vi "Keyence handler_EIP.vi"(8 "error in (no error)":errorcluster, 11 "Message Queues out":T4) -> (0 "error out":errorcluster, 3 "Message Queue":refnum<queue>)   [LabVIEW 2014]
uses:
  support/Message Queue/Message Queue.lvlib
  support/Message Queue/Enqueue Message (Single).vi
  <vilib>/ErrorRing/Error Ring.xnode
  support/Message Queue/Lossy Enqueue Message (Single).vi
  Keyence data cluster_EIP.ctl
  <vilib>/ethernetip/ethernetip.lvlib
  <vilib>/Utility/error.llb/Error Cluster From Error Code.vi
  <vilib>/ethernetip/ethernetip.llb/ethernetip.ctl
  <vilib>/ethernetip/ethernetip.llb/EthernetIPAssemblyType.ctl
  <vilib>/ethernetip/ethernetip.llb/EthernetIP Tag Write BOOL.vi
  Control_EIP.ctl
  Status_EIP.ctl
  support/Message Queue/Message Cluster.ctl
  support/Message Queue/All Message Queues.ctl
panel:
  in  "Inst 2":i32=1
  in  "Inst":i32=1
  in  "Class":i32=1
  in  "Class 2":i32=1
  in  "Attribute 2":i32=1
  in  "Attribute":i32=1
  out "Keyence Data Cluster":T1
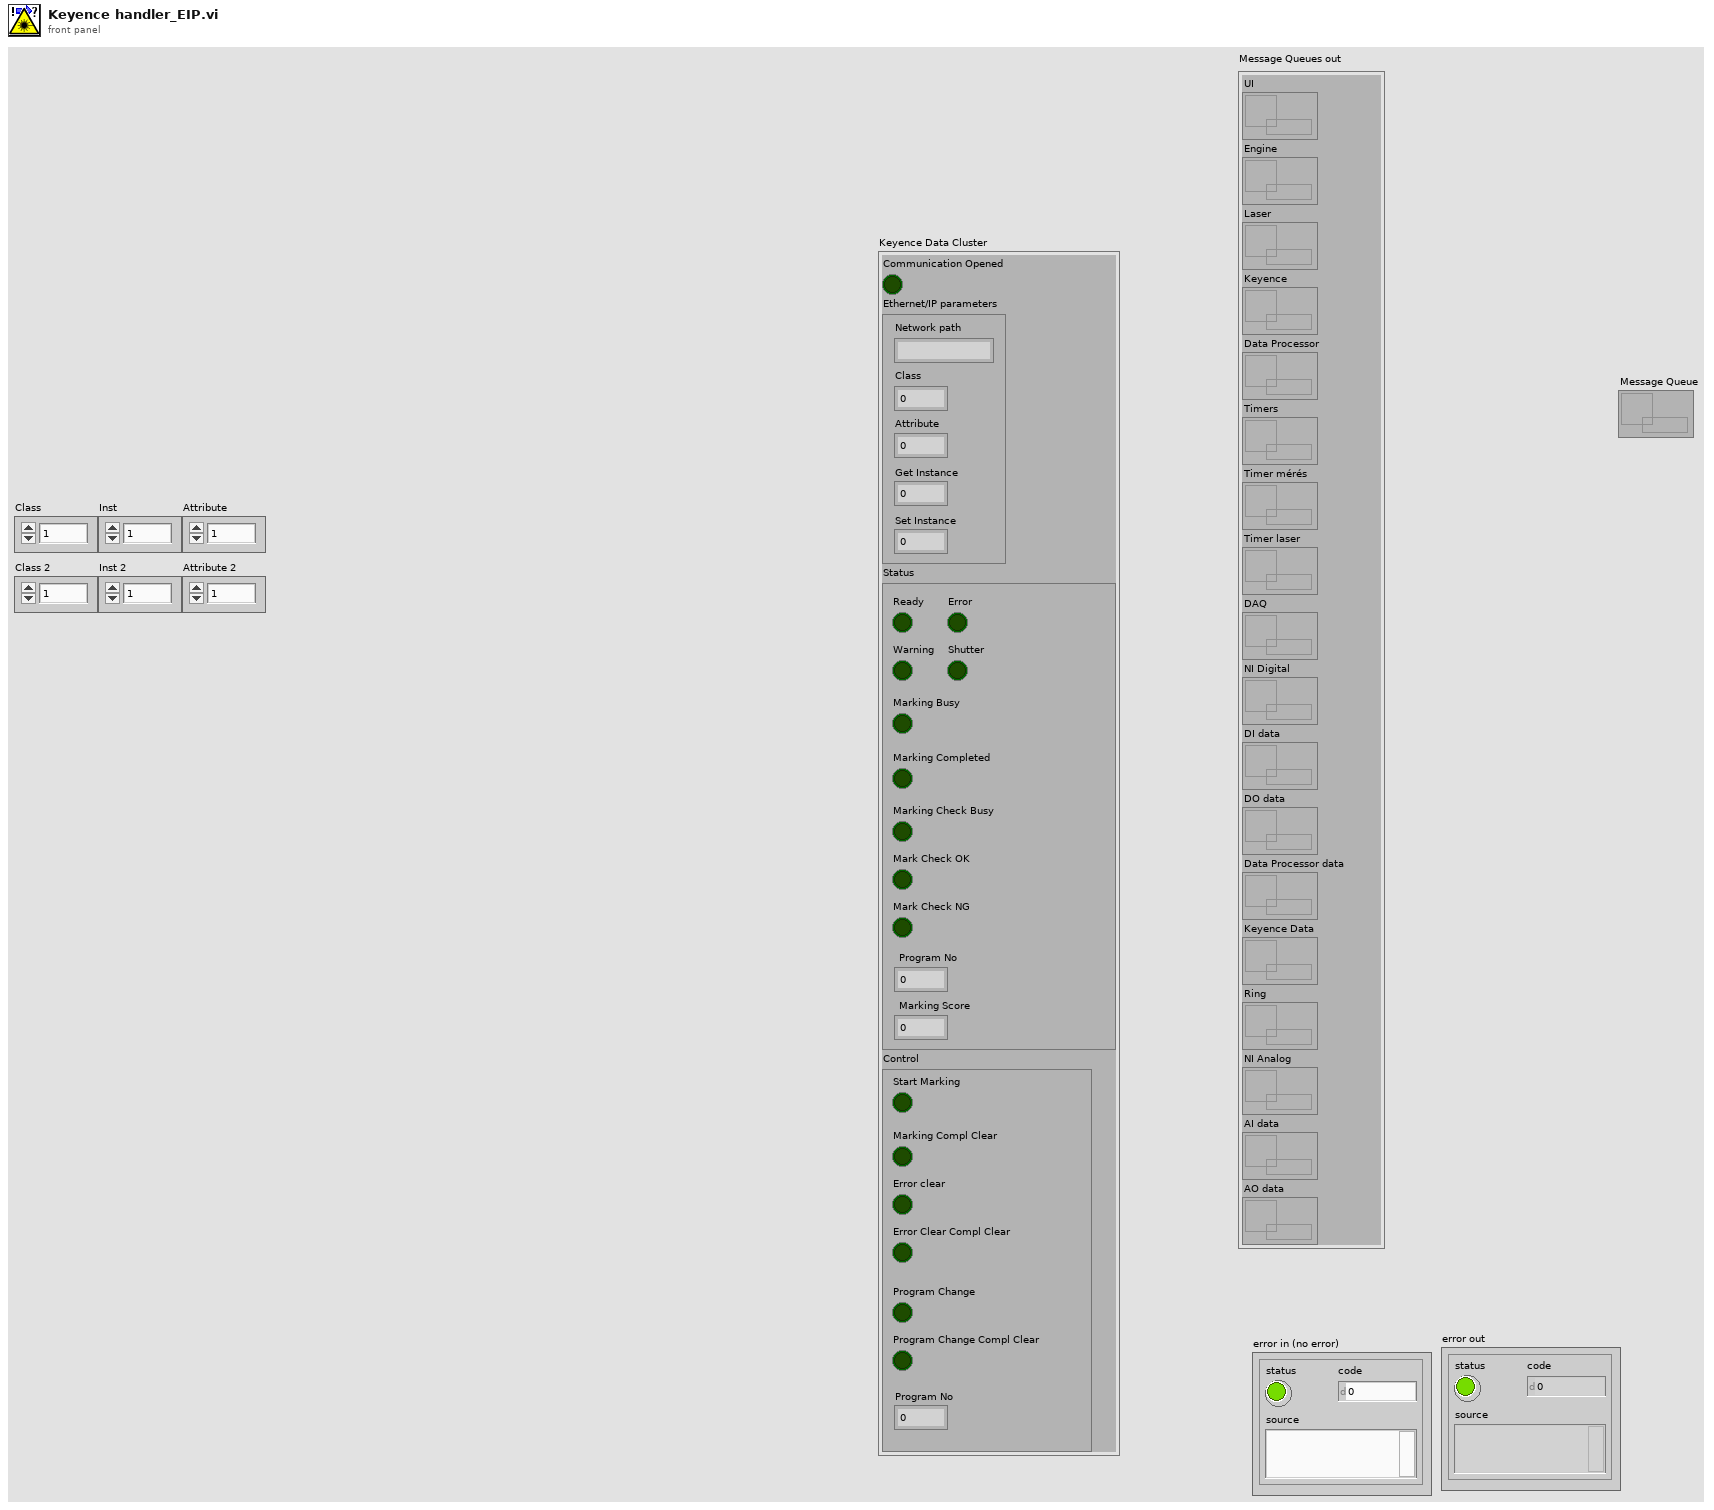
[diagram p1: front panel]
types:
  T1 = typedef "Keyence data cluster_EIP.ctl" = cluster{"Communication Opened":bool, "Ethernet/IP parameters":cluster{"Class":dbl, "Attribute":dbl, "Get Instance":dbl, "Set Instance":dbl, "Network path":string}, "Status":T2, "Control":T3}
  T2 = typedef "Status_EIP.ctl" = cluster{"Ready":bool, "Error":bool, "Warning":bool, "Shutter":bool, "Mark Check OK":bool, "Mark Check NG":bool, "Marking Busy":bool, "Program No":u16, "Marking Check Busy":bool, "Marking Completed":bool, "Marking Score":u16}
  T3 = typedef "Control_EIP.ctl" = cluster{"Start Marking":bool, "Error clear":bool, "Program Change":bool, "Marking Compl Clear":bool, "Program No":u16, "Error Clear Compl Clear":bool, "Program Change Compl Clear":bool}
  T4 = typedef "Message Queue.lvlib/All Message Queues.ctl" = cluster{"UI":refnum<queue>, "Engine":refnum<queue>, "Laser":refnum<queue>, "Keyence":refnum<queue>, "Data Processor":refnum<queue>, "Timers":refnum<queue>, "Timer mérés":refnum<queue>, "Timer laser":refnum<queue>, "DAQ":refnum<queue>, "NI Digital":refnum<queue>, "DI data":refnum<queue>, "DO data":refnum<queue>, "Data Processor data":refnum<queue>, "Keyence Data":refnum<queue>, "Ring":refnum<queue>, "NI Analog":refnum<queue>, "AI data":refnum<queue>, "AO data":refnum<queue>}
  T5 = typedef "ethernetip.lvlib/ethernetip.ctl" = refnum<k21>
  T6 = typedef "ethernetip.lvlib/EthernetIPAssemblyType.ctl" = enum16{"Producing", "Consuming", "Configuration"}
  T7 = typedef "Status.ctl" = cluster{"Ready":bool, "Error":bool, "Warning":bool, "Shutter":bool, "Mark Check OK":bool, "Mark Check NG":bool, "Marking Busy":bool, "Program No":u16, "Marking Check Busy":bool, "Marking Completed":bool, "Marking Score":u16, "Marking Error":bool, "Marking Stop":bool, "Program is changing":bool, "Date/Time":timestamp}
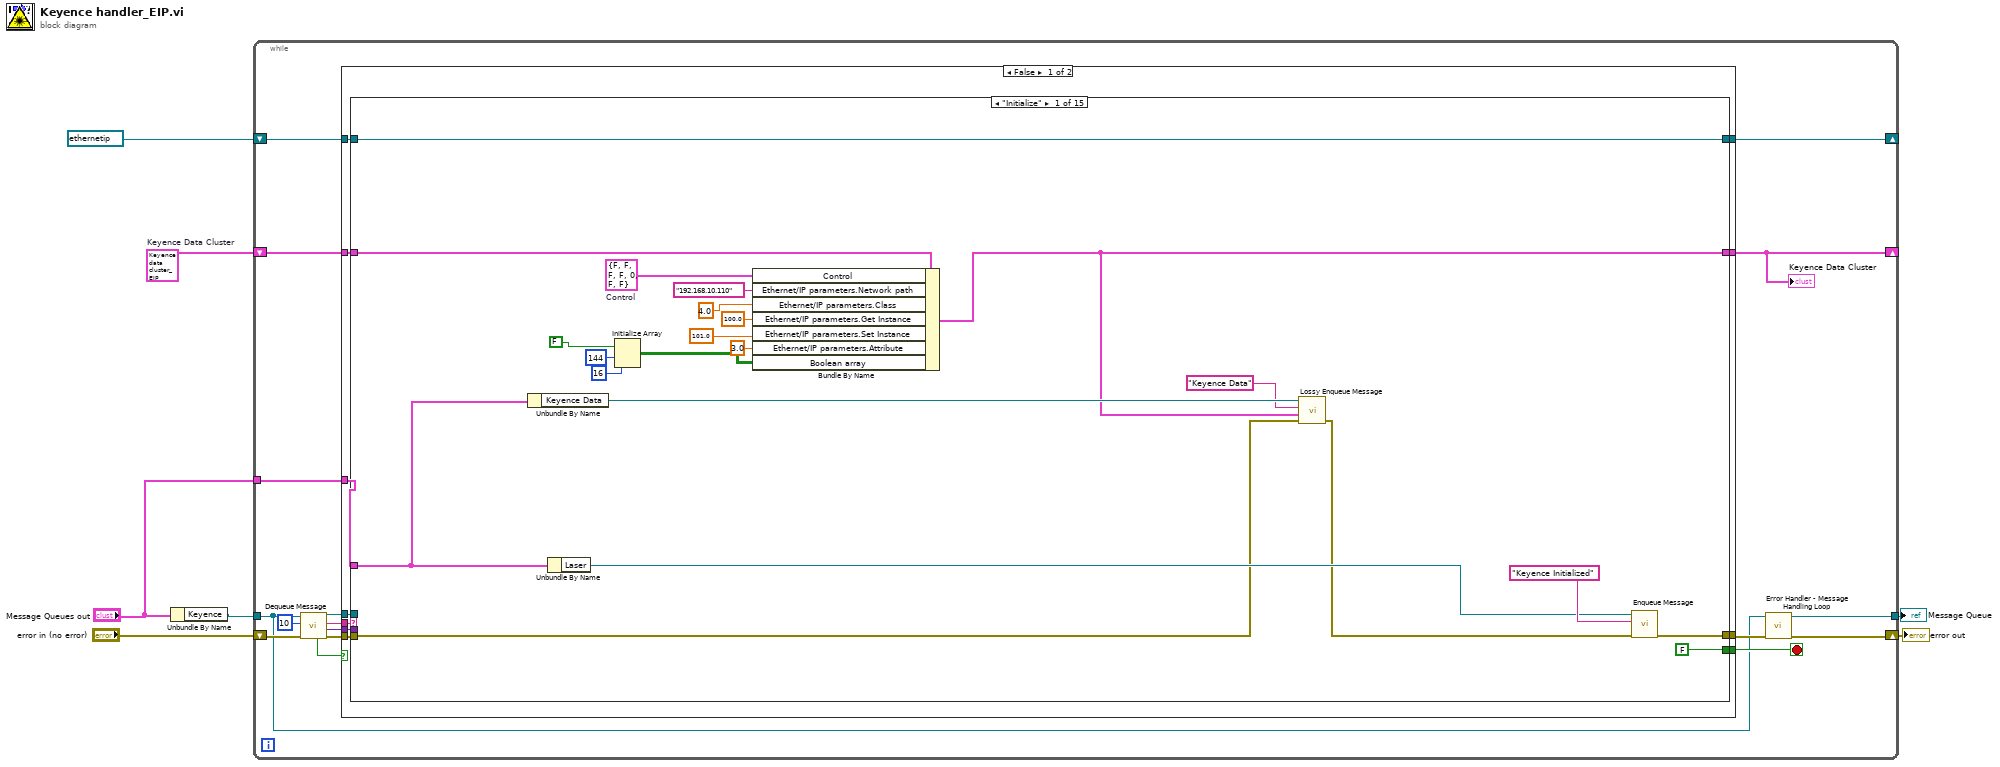
[diagram p0: block diagram]
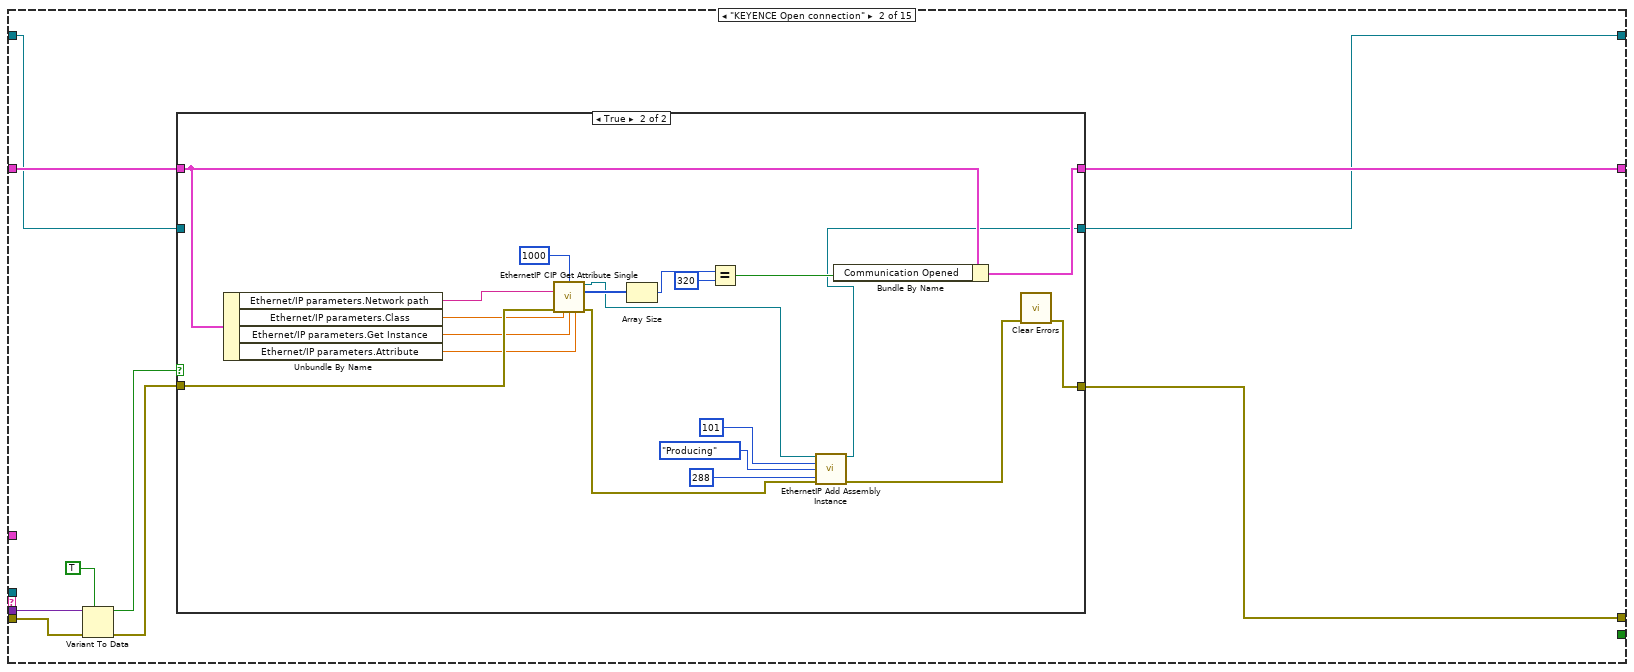
[diagram p2: hidden frame]
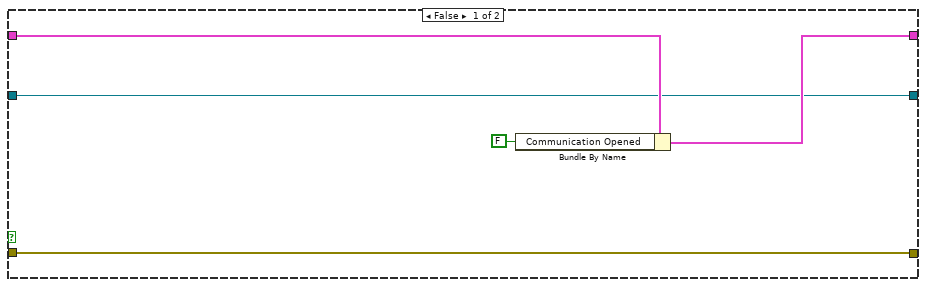
[diagram p3: hidden frame]
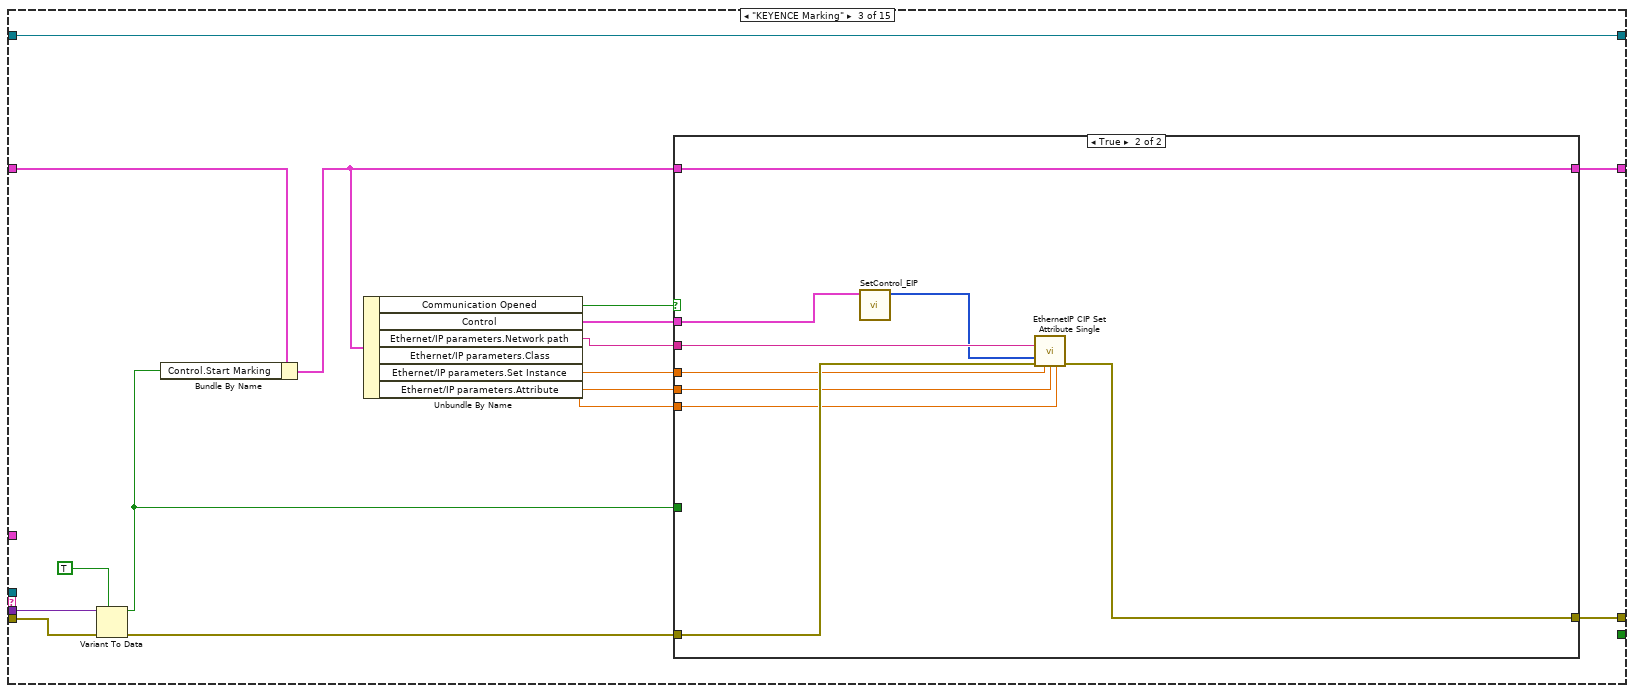
[diagram p4: hidden frame]
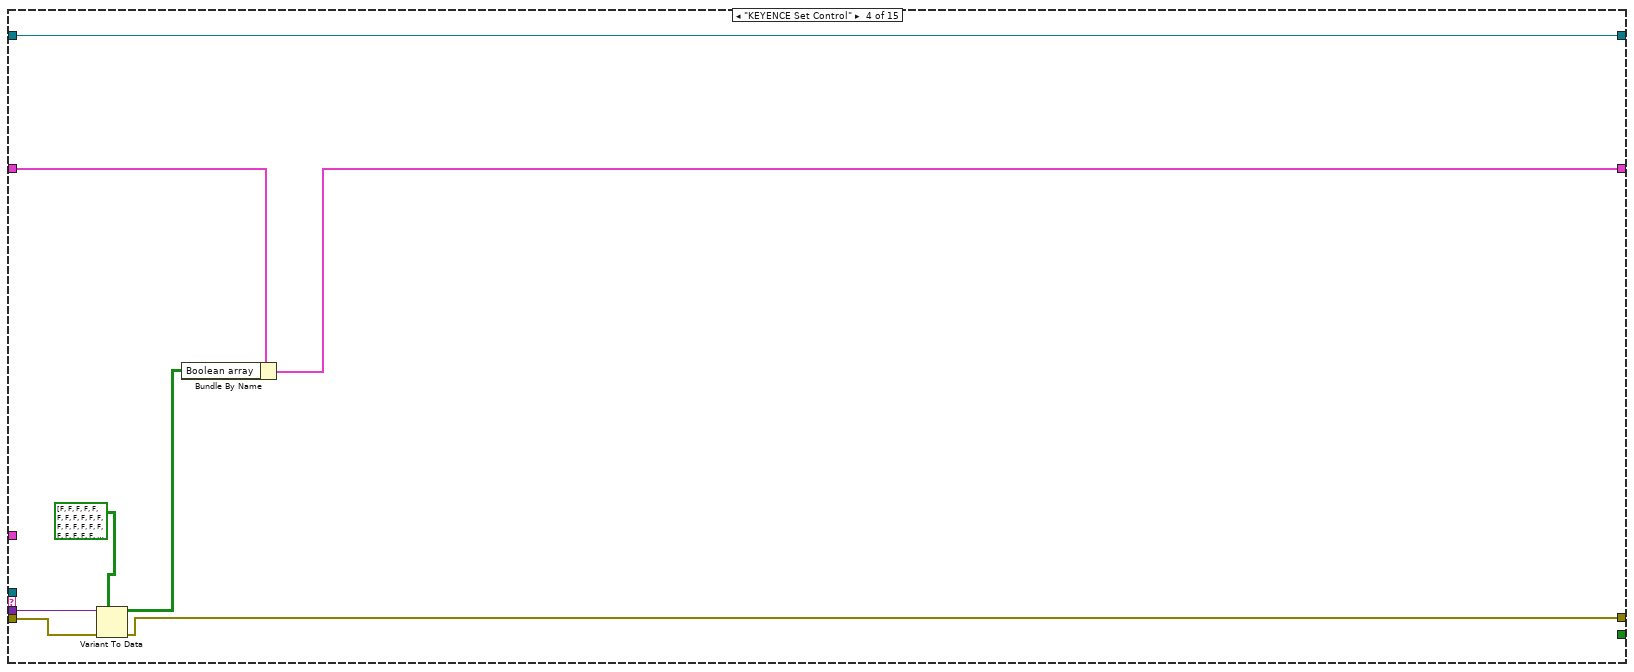
[diagram p6: hidden frame]
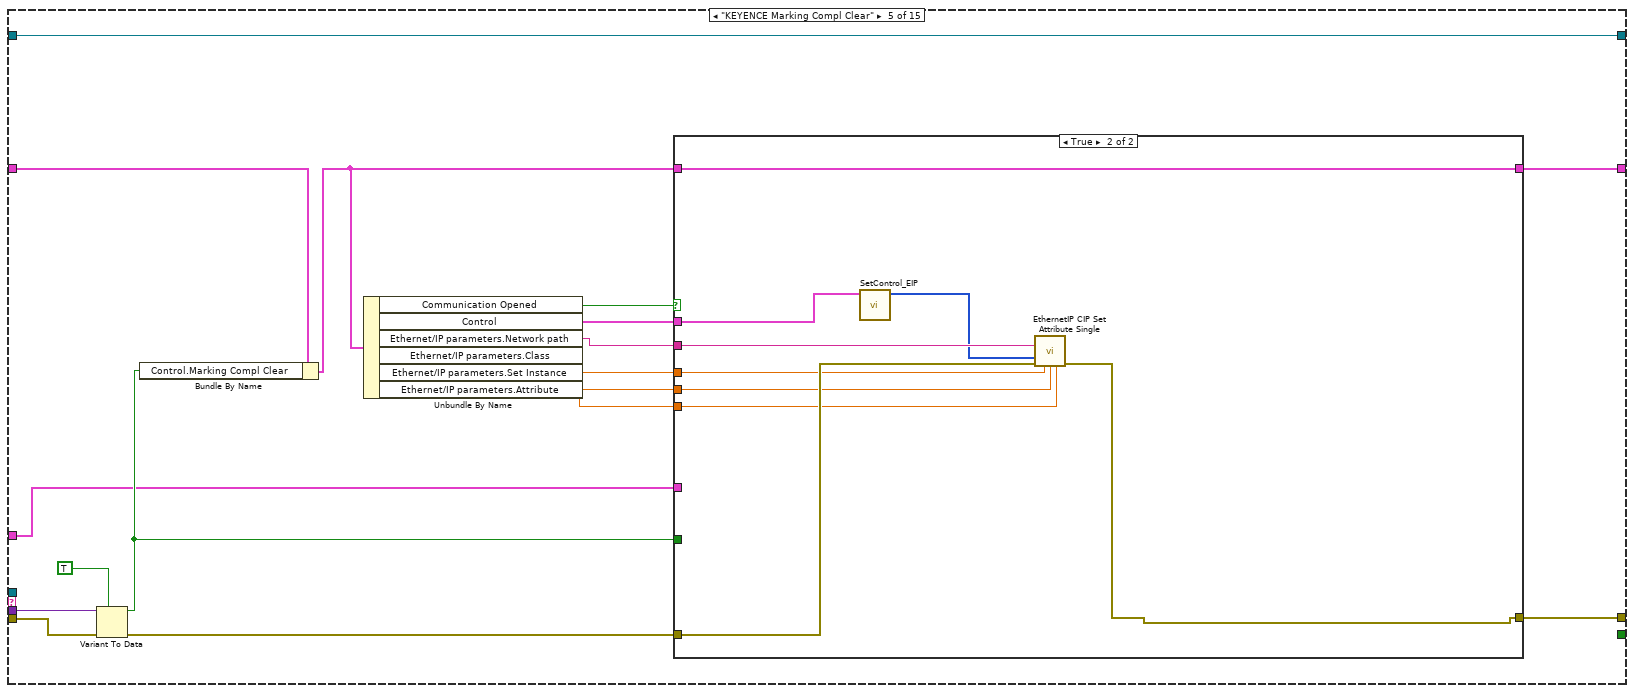
[diagram p7: hidden frame]
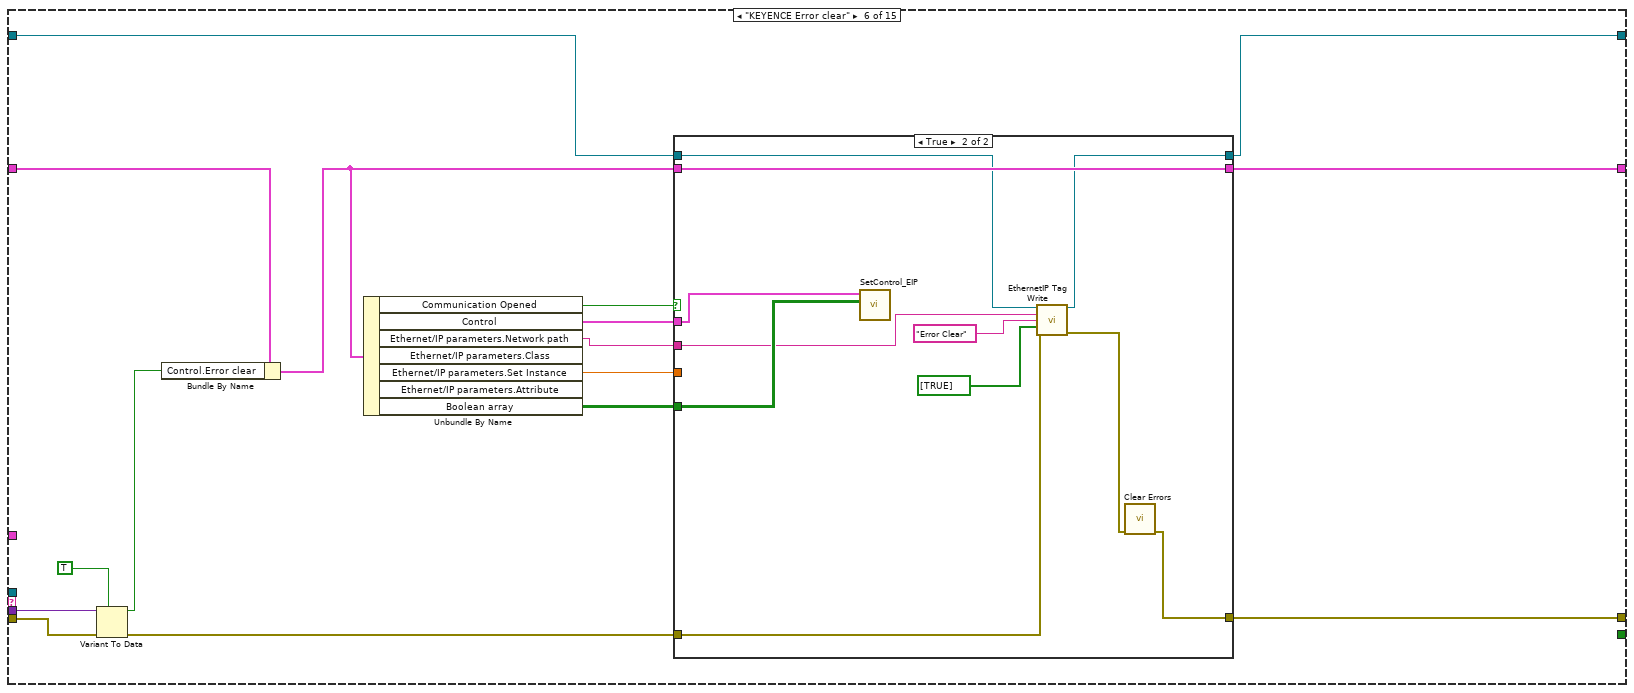
[diagram p9: hidden frame]
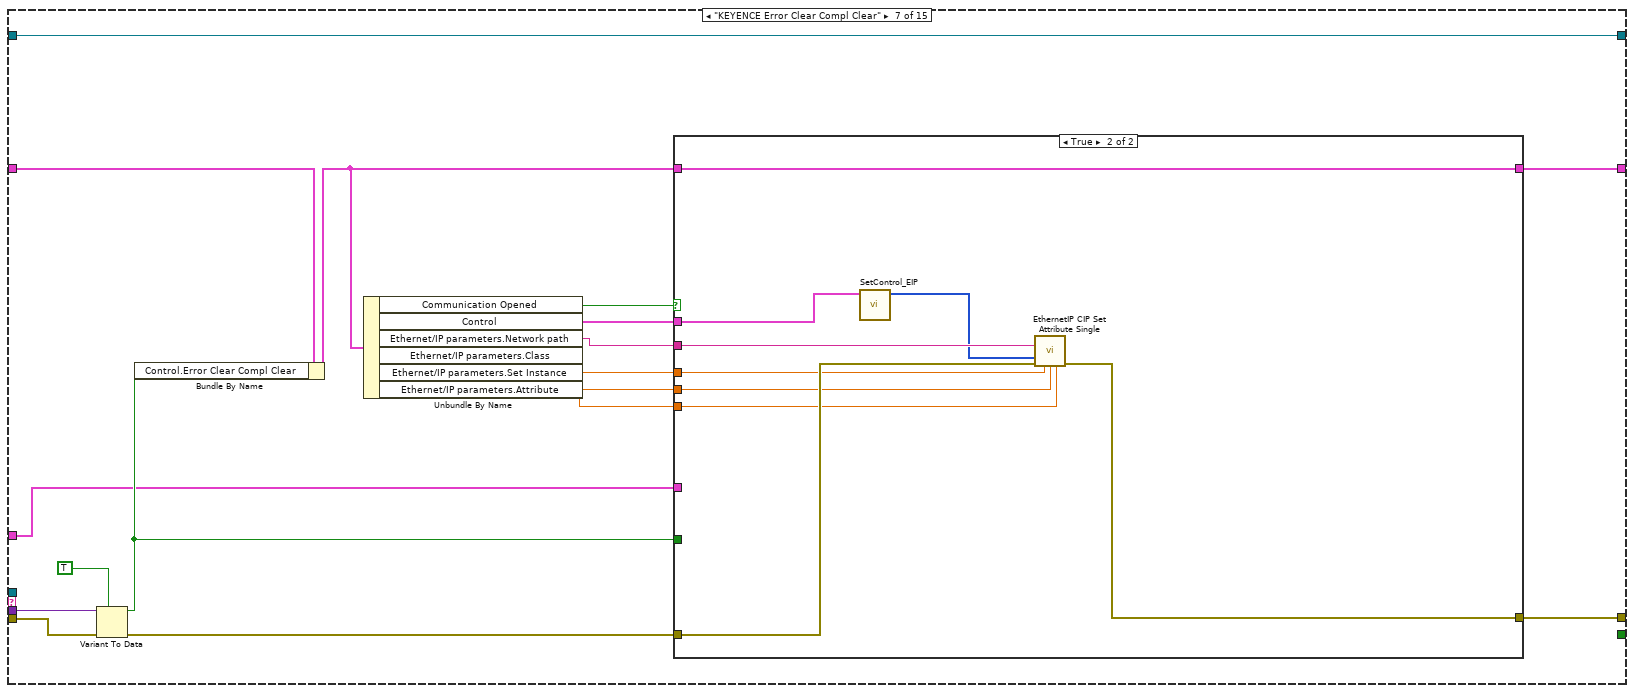
[diagram p11: hidden frame]
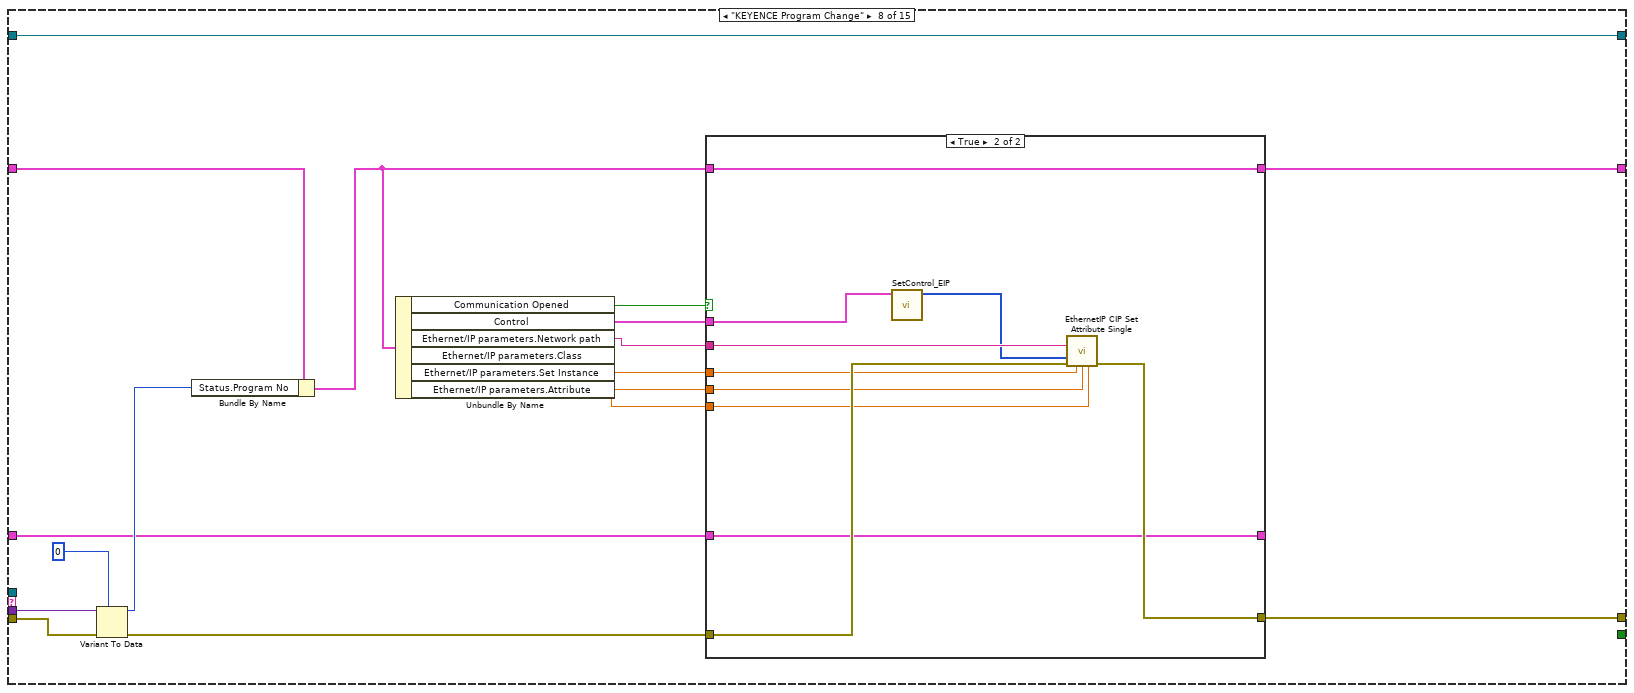
[diagram p13: hidden frame]
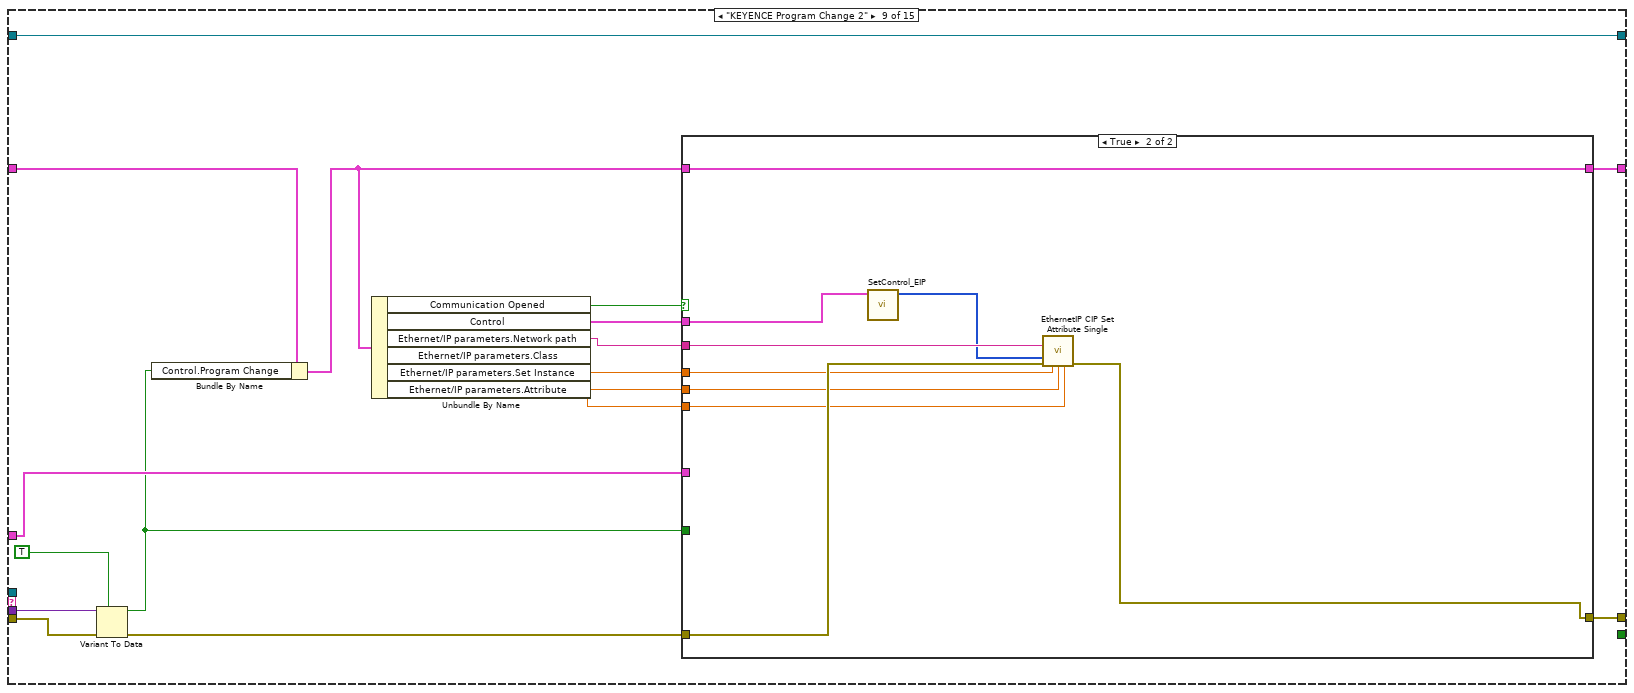
[diagram p15: hidden frame]
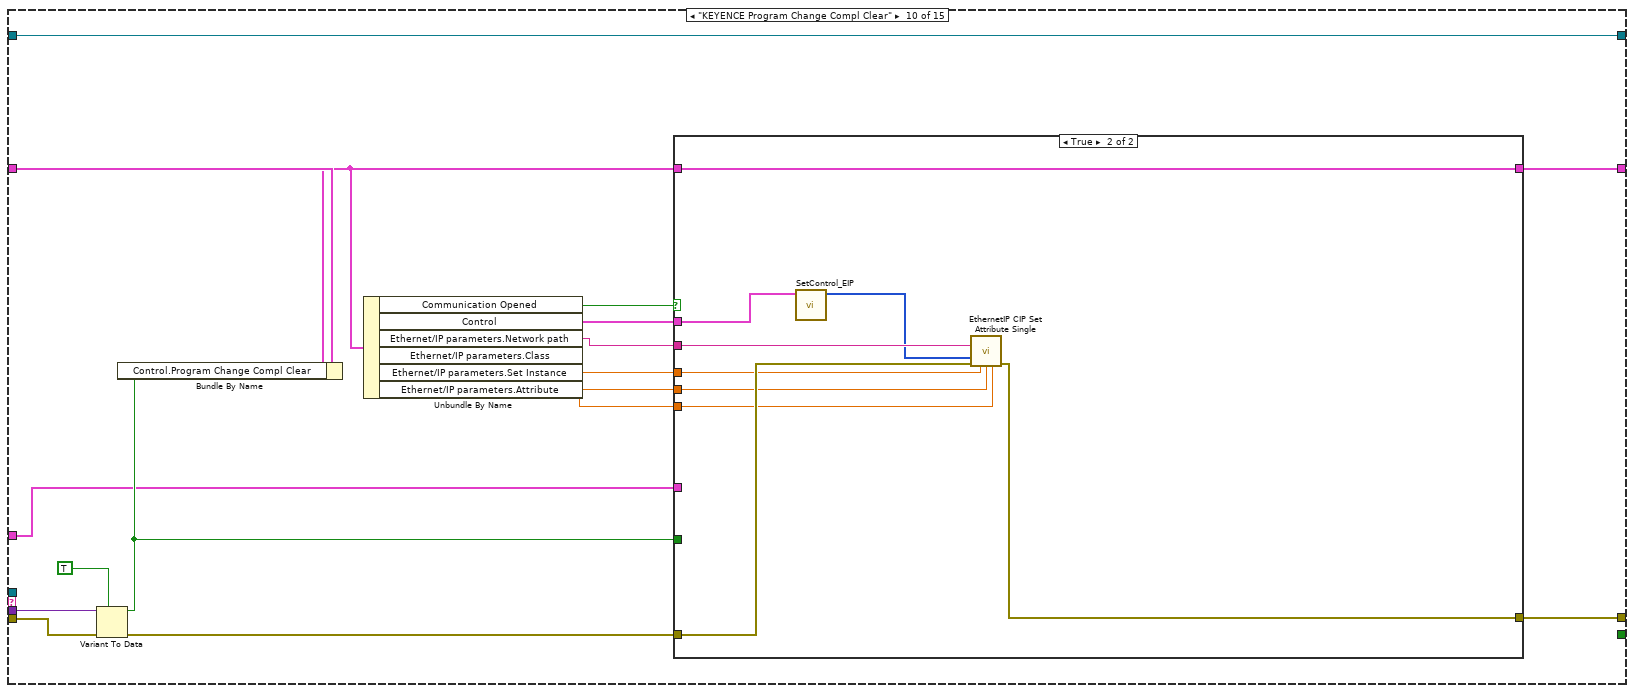
[diagram p17: hidden frame]
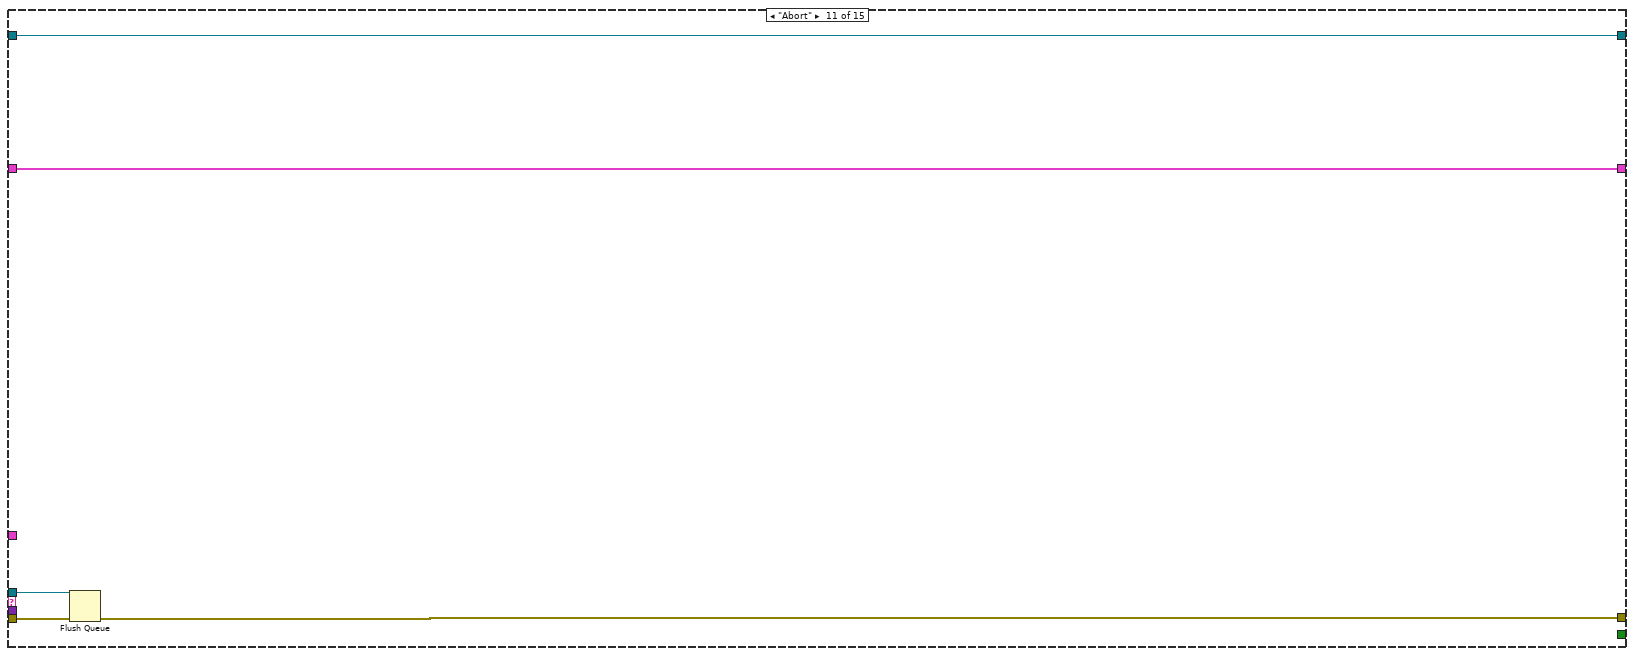
[diagram p19: hidden frame]
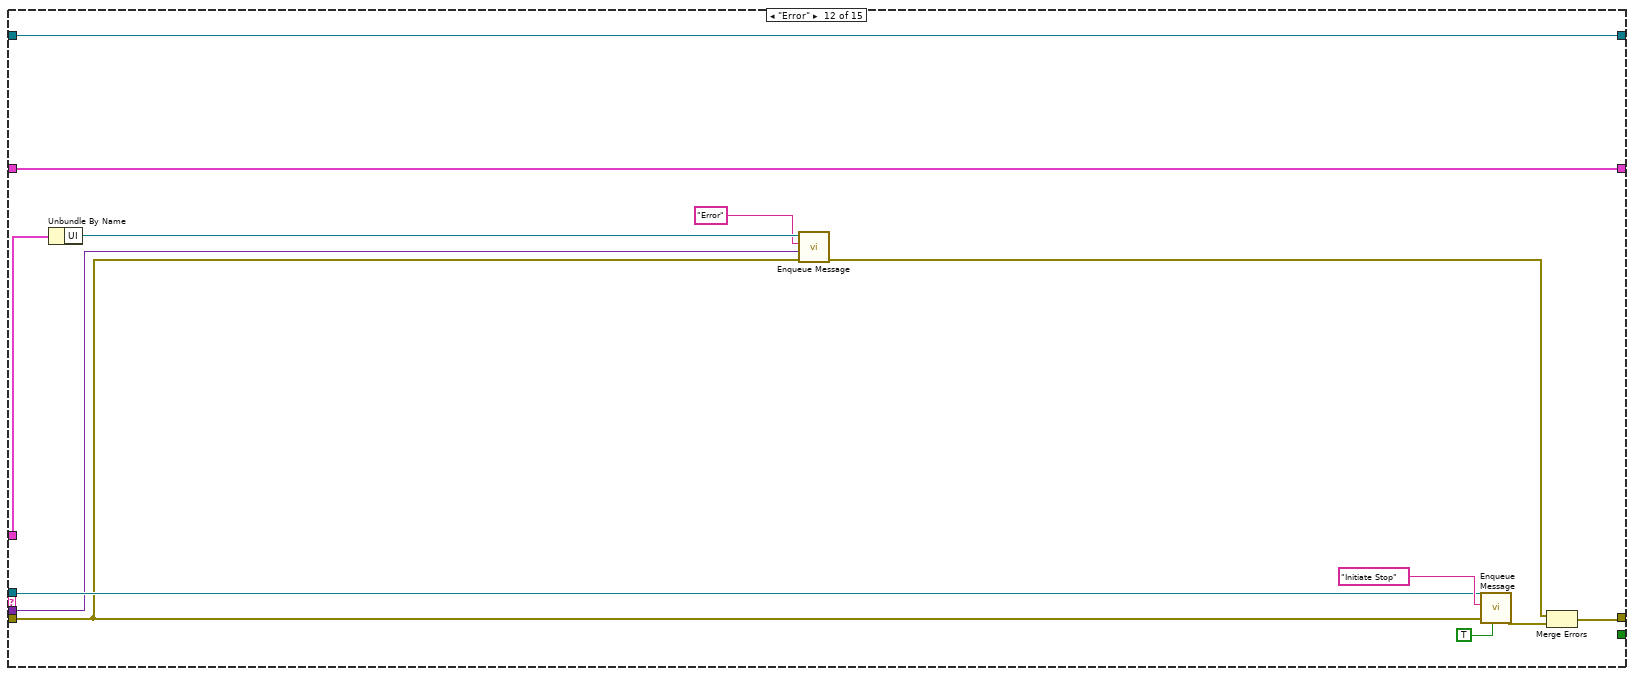
[diagram p20: hidden frame]
diagram:
  w2 = T1 {"Communication Opened"=FALSE, "Ethernet/IP parameters"={"Class"=0.0, "Attribute"=0.0, "Get Instance"=0.0, "Set Instance"=0.0, "Network path"=""}, "Status"={"Ready"=FALSE, "Error"=FALSE, "Warning"=FALSE, "Shutter"=FALSE, "Mark Check OK"=FALSE, "Mark Check NG"=FALSE, "Marking Busy"=FALSE, "Program No"=0, "Marking Check Busy"=FALSE, "Marking Completed"=FALSE, "Marking Score"=0}, "Control"={"Start Marking"=FALSE, "Error clear"=FALSE, "Program Change"=FALSE, "Marking Compl Clear"=FALSE, "Program No"=0, "Error Clear Compl Clear"=FALSE, "Program Change Compl Clear"=FALSE}}  # Keyence Data Cluster
  n1 = Unbundle By Name("Message Queues out") -> ("Keyence"=w4:refnum<queue>)
  n2 = while {
    tunnel: w4 -> [w11]
    shift-right: [w10] -> _
    shift-left: w2 -> [w17]
    shift-right: [w15] -> w7
    shift-left: "error in (no error)" -> [w24]
    tunnel: "Message Queues out" -> [w13]
    tunnel: [w12] -> w3
    shift-right: [w9] -> _
    shift-left: T5 "Default" ("Session in") -> [w8]
    stop <- w20 stop-if-true
    n3 = call "Dequeue Message.vi"("error in (no error)"=w24, "timeout in ms (-1)"=10, "Message Queue"=w11) -> ("error out"=w22:errorcluster, "Message Data"=w16:variant, "Message"=w23:string, "dup Message Queue"=w21:refnum<queue>, "timed out?"=w18:bool)  [unwired: 4 in]
    n4 = case shown="False" w18 {
      tunnel: w23 -> [w35 _]
      tunnel: w22 -> [w34 w363]
      tunnel: w21 -> [w33 _]
      tunnel: [w32 FALSE] -> w20
      tunnel: [w31 w364] -> w14
      tunnel: w17 -> [w30 w362]
      tunnel: [w27 w354] -> w10
      tunnel: w16 -> [w29 _]
      tunnel: w13 -> [w28 w356]
      tunnel: [w26 w349] -> w9
      tunnel: w8 -> [w25 w350]
      frame False {
        n5 = case shown="\"Initialize\"" w35 {
          selector: w35 -> [_ _ _ _ _ _ _ _ _ _ _ _ _ _ w338]
          tunnel: w34 -> [w46 w63 w107 w126 w143 w170 w201 w229 w259 w287 w304 w307 w322 w326 _]
          tunnel: w33 -> [_ _ _ _ _ _ _ _ _ _ w303 w310 w321 w336 _]
          tunnel: [w56 w60 w105 w122 w141 w168 w199 w215 w258 w285 w301 w311 w323 w327 w339] -> w31
          tunnel: [FALSE _ _ _ _ _ _ _ _ _ _ _ _ TRUE FALSE] -> w32
          tunnel: w30 -> [w53 w62 w98 w125 w134 w162 w192 w222 w251 w278 w302 w306 w324 w334 w341]
          tunnel: w29 -> [_ w64 w108 w127 w144 w171 w202 w230 w260 w288 _ w308 _ _ _]
          tunnel: w28 -> [w50 _ _ _ w129 _ w187 w216 w246 w273 _ w309 _ w329 _]
          tunnel: [w47 w61 w95 w121 w131 w159 w189 w219 w248 w275 w302 w306 w324 w334 w341] -> w27
          tunnel: [w36 w59 w93 w120 w128 w157 w186 w214 w244 w272 w300 w305 w318 w325 w337] -> w26
          tunnel: w25 -> [w36 w58 w93 w120 w128 w158 w186 w214 w244 w272 w300 w305 w318 w325 w337]
          frame "Initialize" {
            w52 = T3 {"Start Marking"=FALSE, "Error clear"=FALSE, "Program Change"=FALSE, "Marking Compl Clear"=FALSE, "Program No"=0, "Error Clear Compl Clear"=FALSE, "Program Change Compl Clear"=FALSE}  # Control
            n6 = Unbundle By Name(w50) -> ("Keyence Data"=w49:refnum<queue>)
            n7 = Unbundle By Name(w50) -> ("Laser"=w54:refnum<queue>)
            n8 = Initialize Array(FALSE, 144 ("dimension size"), 16 ("dimension size")) -> (w38:bool[][])
            n9 = Bundle By Name(cluster=w53, "Control"=w52, "Ethernet/IP parameters.Network path"="192.168.10.110", "Ethernet/IP parameters.Class"=4.0, "Ethernet/IP parameters.Get Instance"=100.0, "Ethernet/IP parameters.Set Instance"=101.0, "Ethernet/IP parameters.Attribute"=3.0, "Boolean array"=w38) -> (w47:T1)
            n10 = call-poly "Lossy Enqueue Message.vi"("error in (no error)"=w46, "Message Data"=w47, "Message"="Keyence Data", "Message Queue"=w49) -> ("error out"=w45:errorcluster)  [unwired: 6 in, 1 out]
            n11 = call-poly "Enqueue Message.vi"("error in (no error)"=w45, "Message"="Keyence Initialized", "Message Queue"=w54) -> ("error out"=w56:errorcluster)  [unwired: 7 in, 1 out]
          }
          frame "KEYENCE Open connection" {
            n12 = Variant To Data(error in=w63, type=TRUE ("Control word.Enable Voltage"), Variant=w64) -> (data=w65:bool, error out=w66:errorcluster)
            n13 = case shown="True" w65 {
              tunnel: w66 -> [w69 w92]
              tunnel: w62 -> [w72 w91]
              tunnel: [w69 w81] -> w60
              tunnel: [w70 w90] -> w61
              tunnel: [w68 w73] -> w59
              tunnel: w58 -> [w68 _]
              frame False {
                n14 = Bundle By Name(cluster=w72, "Communication Opened"=FALSE) -> (w70:T1)
              }
              frame True {
                n15 = Unbundle By Name(w91) -> ("Ethernet/IP parameters.Network path"=w89:string, "Ethernet/IP parameters.Class"=w88:dbl, "Ethernet/IP parameters.Get Instance"=w86:dbl, "Ethernet/IP parameters.Attribute"=w87:dbl)
                n16 = call <vilib>:"EthernetIP CIP Get Attribute Single.vi"("Timeout (ms)"=1000, "Network Path"=w89, "error in"=w92, "Class"=w88, "Instance"=w86, "Attribute"=w87) -> ("Session out"=w74:T5, "Data"=w85:u8[], "error out"=w76:errorcluster)  [unwired: 7 in]
                n17 = Array Size(array=w85) -> (size(s)=w83:i32)
                n18 = Equal?(x=w83, y=320) -> (x = y?=w84:bool)
                n19 = call <vilib>:"EthernetIP Add Assembly Instance.vi"("Session in"=w74, "Instance ID in"=u32 101, "Type"=EthernetIPAssemblyType."Producing", "Size (bytes)"=u32 288, "error in"=w76) -> ("Session out"=w73:T5, "error out"=w77:errorcluster)  [unwired: 8 in, 1 out]
                n20 = Bundle By Name(cluster=w91, "Communication Opened"=w84) -> (w90:T1)
                n21 = call <vilib>:"Clear Errors.vi"("error in (no error)"=w77) -> ("error out"=w81:errorcluster)  [unwired: 5 in, 1 out]
              }
            }
          }
          frame "KEYENCE Marking" {
            n22 = Variant To Data(error in=w107, type=TRUE, Variant=w108) -> (data=w94:bool, error out=w104:errorcluster)
            n23 = Bundle By Name(cluster=w98, "Control.Start Marking"=w94) -> (w96:T1)
            n24 = Unbundle By Name(w96) -> ("Communication Opened"=w97:bool, "Control"=w99:T3, "Ethernet/IP parameters.Network path"=w103:string, "Ethernet/IP parameters.Class"=w102:dbl, "Ethernet/IP parameters.Set Instance"=w101:dbl, "Ethernet/IP parameters.Attribute"=w100:dbl)
            n25 = case shown="True" w97 {
              tunnel: [w109 w111] -> w105
              tunnel: w104 -> [w109 w119]
              tunnel: w103 -> [_ w118]
              tunnel: w102 -> [_ w117]
              tunnel: w101 -> [_ w116]
              tunnel: w100 -> [_ w115]
              tunnel: w99 -> [_ w114]
              tunnel: w96 -> [w110 w112]
              tunnel: [w110 w112] -> w95
              tunnel: w94 -> [_ _]
              frame False {
              }
              frame True {
                n26 = call "SetControl_EIP.vi"("variant"=w114) -> ("Data"=w113:u8[])  [unwired: 10 in]
                n27 = call <vilib>:"EthernetIP CIP Set Attribute Single.vi"("Network Path"=w118, "Data"=w113, "error in"=w119, "Class"=w117, "Instance"=w116, "Attribute"=w115) -> ("error out"=w111:errorcluster)  [unwired: 8 in, 1 out]
              }
            }
          }
          frame "KEYENCE Set Control" {
            n28 = Variant To Data(error in=w126, type=bool[][] [[FALSE, FALSE, FALSE, FALSE, FALSE, FALSE, FALSE, FALSE, FALSE, FALSE, FALSE, FALSE, FALSE, FALSE, FALSE, FALSE], [FALSE, FALSE, FALSE, FALSE, FALSE, FALSE, FALSE, FALSE, FALSE, FALSE, FALSE, FALSE, FALSE, FALSE, FALSE, FALSE], [FALSE, FALSE, FALSE, FALSE, FALSE, FALSE, FALSE, FALSE, FALSE, FALSE, FALSE, FALSE, FALSE, FALSE, FALSE, FALSE], [FALSE, FALSE, FALSE, FALSE, FALSE, FALSE, FALSE, FALSE, FALSE, FALSE, FALSE, FALSE, FALSE, FALSE, FALSE, FALSE], [FALSE, FALSE, FALSE, FALSE, FALSE, FALSE, FALSE, FALSE, FALSE, FALSE, FALSE, FALSE, FALSE, FALSE, FALSE, FALSE], [FALSE, FALSE, FALSE, FALSE, FALSE, FALSE, FALSE, FALSE, FALSE, FALSE, FALSE, FALSE, FALSE, FALSE, FALSE, FALSE], [FALSE, FALSE, FALSE, FALSE, FALSE, FALSE, FALSE, FALSE, FALSE, FALSE, FALSE, FALSE, FALSE, FALSE, FALSE, FALSE], [FALSE, FALSE, FALSE, FALSE, FALSE, FALSE, FALSE, FALSE, FALSE, FALSE, FALSE, FALSE, FALSE, FALSE, FALSE, FALSE], [FALSE, FALSE, FALSE, FALSE, FALSE, FALSE, FALSE, FALSE, FALSE, FALSE, FALSE, FALSE, FALSE, FALSE, FALSE, FALSE], [FALSE, FALSE, FALSE, FALSE, FALSE, FALSE, FALSE, FALSE, FALSE, FALSE, FALSE, FALSE, FALSE, FALSE, FALSE, FALSE], [FALSE, FALSE, FALSE, FALSE, FALSE, FALSE, FALSE, FALSE, FALSE, FALSE, FALSE, FALSE, FALSE, FALSE, FALSE, FALSE], [FALSE, FALSE, FALSE, FALSE, FALSE, FALSE, FALSE, FALSE, FALSE, FALSE, FALSE, FALSE, FALSE, FALSE, FALSE, FALSE], [FALSE, FALSE, FALSE, FALSE, FALSE, FALSE, FALSE, FALSE, FALSE, FALSE, FALSE, FALSE, FALSE, FALSE, FALSE, FALSE], [FALSE, FALSE, FALSE, FALSE, FALSE, FALSE, FALSE, FALSE, FALSE, FALSE, FALSE, FALSE, FALSE, FALSE, FALSE, FALSE], [FALSE, FALSE, FALSE, FALSE, FALSE, FALSE, FALSE, FALSE, FALSE, FALSE, FALSE, FALSE, FALSE, FALSE, FALSE, FALSE], [FALSE, FALSE, FALSE, FALSE, FALSE, FALSE, FALSE, FALSE, FALSE, FALSE, FALSE, FALSE, FALSE, FALSE, FALSE, FALSE], [FALSE, FALSE, FALSE, FALSE, FALSE, FALSE, FALSE, FALSE, FALSE, FALSE, FALSE, FALSE, FALSE, FALSE, FALSE, FALSE], [FALSE, FALSE, FALSE, FALSE, FALSE, FALSE, FALSE, FALSE, FALSE, FALSE, FALSE, FALSE, FALSE, FALSE, FALSE, FALSE], [FALSE, FALSE, FALSE, FALSE, FALSE, FALSE, FALSE, FALSE, FALSE, FALSE, FALSE, FALSE, FALSE, FALSE, FALSE, FALSE], [FALSE, FALSE, FALSE, FALSE, FALSE, FALSE, FALSE, FALSE, FALSE, FALSE, FALSE, FALSE, FALSE, FALSE, FALSE, FALSE], [FALSE, FALSE, FALSE, FALSE, FALSE, FALSE, FALSE, FALSE, FALSE, FALSE, FALSE, FALSE, FALSE, FALSE, FALSE, FALSE], [FALSE, FALSE, FALSE, FALSE, FALSE, FALSE, FALSE, FALSE, FALSE, FALSE, FALSE, FALSE, FALSE, FALSE, FALSE, FALSE], [FALSE, FALSE, FALSE, FALSE, FALSE, FALSE, FALSE, FALSE, FALSE, FALSE, FALSE, FALSE, FALSE, FALSE, FALSE, FALSE], [FALSE, FALSE, FALSE, FALSE, FALSE, FALSE, FALSE, FALSE, FALSE, FALSE, FALSE, FALSE, FALSE, FALSE, FALSE, FALSE], [FALSE, FALSE, FALSE, FALSE, FALSE, FALSE, FALSE, FALSE, FALSE, FALSE, FALSE, FALSE, FALSE, FALSE, FALSE, FALSE], [FALSE, FALSE, FALSE, FALSE, FALSE, FALSE, FALSE, FALSE, FALSE, FALSE, FALSE, FALSE, FALSE, FALSE, FALSE, FALSE], [FALSE, FALSE, FALSE, FALSE, FALSE, FALSE, FALSE, FALSE, FALSE, FALSE, FALSE, FALSE, FALSE, FALSE, FALSE, FALSE], [FALSE, FALSE, FALSE, FALSE, FALSE, FALSE, FALSE, FALSE, FALSE, FALSE, FALSE, FALSE, FALSE, FALSE, FALSE, FALSE], [FALSE, FALSE, FALSE, FALSE, FALSE, FALSE, FALSE, FALSE, FALSE, FALSE, FALSE, FALSE, FALSE, FALSE, FALSE, FALSE], [FALSE, FALSE, FALSE, FALSE, FALSE, FALSE, FALSE, FALSE, FALSE, FALSE, FALSE, FALSE, FALSE, FALSE, FALSE, FALSE], [FALSE, FALSE, FALSE, FALSE, FALSE, FALSE, FALSE, FALSE, FALSE, FALSE, FALSE, FALSE, FALSE, FALSE, FALSE, FALSE], [FALSE, FALSE, FALSE, FALSE, FALSE, FALSE, FALSE, FALSE, FALSE, FALSE, FALSE, FALSE, FALSE, FALSE, FALSE, FALSE], [FALSE, FALSE, FALSE, FALSE, FALSE, FALSE, FALSE, FALSE, FALSE, FALSE, FALSE, FALSE, FALSE, FALSE, FALSE, FALSE], [FALSE, FALSE, FALSE, FALSE, FALSE, FALSE, FALSE, FALSE, FALSE, FALSE, FALSE, FALSE, FALSE, FALSE, FALSE, FALSE], [FALSE, FALSE, FALSE, FALSE, FALSE, FALSE, FALSE, FALSE, FALSE, FALSE, FALSE, FALSE, FALSE, FALSE, FALSE, FALSE], [FALSE, FALSE, FALSE, FALSE, FALSE, FALSE, FALSE, FALSE, FALSE, FALSE, FALSE, FALSE, FALSE, FALSE, FALSE, FALSE], [FALSE, FALSE, FALSE, FALSE, FALSE, FALSE, FALSE, FALSE, FALSE, FALSE, FALSE, FALSE, FALSE, FALSE, FALSE, FALSE], [FALSE, FALSE, FALSE, FALSE, FALSE, FALSE, FALSE, FALSE, FALSE, FALSE, FALSE, FALSE, FALSE, FALSE, FALSE, FALSE], [FALSE, FALSE, FALSE, FALSE, FALSE, FALSE, FALSE, FALSE, FALSE, FALSE, FALSE, FALSE, FALSE, FALSE, FALSE, FALSE], [FALSE, FALSE, FALSE, FALSE, FALSE, FALSE, FALSE, FALSE, FALSE, FALSE, FALSE, FALSE, FALSE, FALSE, FALSE, FALSE], [FALSE, FALSE, FALSE, FALSE, FALSE, FALSE, FALSE, FALSE, FALSE, FALSE, FALSE, FALSE, FALSE, FALSE, FALSE, FALSE], [FALSE, FALSE, FALSE, FALSE, FALSE, FALSE, FALSE, FALSE, FALSE, FALSE, FALSE, FALSE, FALSE, FALSE, FALSE, FALSE], [FALSE, FALSE, FALSE, FALSE, FALSE, FALSE, FALSE, FALSE, FALSE, FALSE, FALSE, FALSE, FALSE, FALSE, FALSE, FALSE], [FALSE, FALSE, FALSE, FALSE, FALSE, FALSE, FALSE, FALSE, FALSE, FALSE, FALSE, FALSE, FALSE, FALSE, FALSE, FALSE], [FALSE, FALSE, FALSE, FALSE, FALSE, FALSE, FALSE, FALSE, FALSE, FALSE, FALSE, FALSE, FALSE, FALSE, FALSE, FALSE], [FALSE, FALSE, FALSE, FALSE, FALSE, FALSE, FALSE, FALSE, FALSE, FALSE, FALSE, FALSE, FALSE, FALSE, FALSE, FALSE], [FALSE, FALSE, FALSE, FALSE, FALSE, FALSE, FALSE, FALSE, FALSE, FALSE, FALSE, FALSE, FALSE, FALSE, FALSE, FALSE], [FALSE, FALSE, FALSE, FALSE, FALSE, FALSE, FALSE, FALSE, FALSE, FALSE, FALSE, FALSE, FALSE, FALSE, FALSE, FALSE], [FALSE, FALSE, FALSE, FALSE, FALSE, FALSE, FALSE, FALSE, FALSE, FALSE, FALSE, FALSE, FALSE, FALSE, FALSE, FALSE], [FALSE, FALSE, FALSE, FALSE, FALSE, FALSE, FALSE, FALSE, FALSE, FALSE, FALSE, FALSE, FALSE, FALSE, FALSE, FALSE], [FALSE, FALSE, FALSE, FALSE, FALSE, FALSE, FALSE, FALSE, FALSE, FALSE, FALSE, FALSE, FALSE, FALSE, FALSE, FALSE], [FALSE, FALSE, FALSE, FALSE, FALSE, FALSE, FALSE, FALSE, FALSE, FALSE, FALSE, FALSE, FALSE, FALSE, FALSE, FALSE], [FALSE, FALSE, FALSE, FALSE, FALSE, FALSE, FALSE, FALSE, FALSE, FALSE, FALSE, FALSE, FALSE, FALSE, FALSE, FALSE], [FALSE, FALSE, FALSE, FALSE, FALSE, FALSE, FALSE, FALSE, FALSE, FALSE, FALSE, FALSE, FALSE, FALSE, FALSE, FALSE], [FALSE, FALSE, FALSE, FALSE, FALSE, FALSE, FALSE, FALSE, FALSE, FALSE, FALSE, FALSE, FALSE, FALSE, FALSE, FALSE], [FALSE, FALSE, FALSE, FALSE, FALSE, FALSE, FALSE, FALSE, FALSE, FALSE, FALSE, FALSE, FALSE, FALSE, FALSE, FALSE], [FALSE, FALSE, FALSE, FALSE, FALSE, FALSE, FALSE, FALSE, FALSE, FALSE, FALSE, FALSE, FALSE, FALSE, FALSE, FALSE], [FALSE, FALSE, FALSE, FALSE, FALSE, FALSE, FALSE, FALSE, FALSE, FALSE, FALSE, FALSE, FALSE, FALSE, FALSE, FALSE], [FALSE, FALSE, FALSE, FALSE, FALSE, FALSE, FALSE, FALSE, FALSE, FALSE, FALSE, FALSE, FALSE, FALSE, FALSE, FALSE], [FALSE, FALSE, FALSE, FALSE, FALSE, FALSE, FALSE, FALSE, FALSE, FALSE, FALSE, FALSE, FALSE, FALSE, FALSE, FALSE], [FALSE, FALSE, FALSE, FALSE, FALSE, FALSE, FALSE, FALSE, FALSE, FALSE, FALSE, FALSE, FALSE, FALSE, FALSE, FALSE], [FALSE, FALSE, FALSE, FALSE, FALSE, FALSE, FALSE, FALSE, FALSE, FALSE, FALSE, FALSE, FALSE, FALSE, FALSE, FALSE], [FALSE, FALSE, FALSE, FALSE, FALSE, FALSE, FALSE, FALSE, FALSE, FALSE, FALSE, FALSE, FALSE, FALSE, FALSE, FALSE], [FALSE, FALSE, FALSE, FALSE, FALSE, FALSE, FALSE, FALSE, FALSE, FALSE, FALSE, FALSE, FALSE, FALSE, FALSE, FALSE], [FALSE, FALSE, FALSE, FALSE, FALSE, FALSE, FALSE, FALSE, FALSE, FALSE, FALSE, FALSE, FALSE, FALSE, FALSE, FALSE], [FALSE, FALSE, FALSE, FALSE, FALSE, FALSE, FALSE, FALSE, FALSE, FALSE, FALSE, FALSE, FALSE, FALSE, FALSE, FALSE], [FALSE, FALSE, FALSE, FALSE, FALSE, FALSE, FALSE, FALSE, FALSE, FALSE, FALSE, FALSE, FALSE, FALSE, FALSE, FALSE], [FALSE, FALSE, FALSE, FALSE, FALSE, FALSE, FALSE, FALSE, FALSE, FALSE, FALSE, FALSE, FALSE, FALSE, FALSE, FALSE], [FALSE, FALSE, FALSE, FALSE, FALSE, FALSE, FALSE, FALSE, FALSE, FALSE, FALSE, FALSE, FALSE, FALSE, FALSE, FALSE], [FALSE, FALSE, FALSE, FALSE, FALSE, FALSE, FALSE, FALSE, FALSE, FALSE, FALSE, FALSE, FALSE, FALSE, FALSE, FALSE], [FALSE, FALSE, FALSE, FALSE, FALSE, FALSE, FALSE, FALSE, FALSE, FALSE, FALSE, FALSE, FALSE, FALSE, FALSE, FALSE], [FALSE, FALSE, FALSE, FALSE, FALSE, FALSE, FALSE, FALSE, FALSE, FALSE, FALSE, FALSE, FALSE, FALSE, FALSE, FALSE], [FALSE, FALSE, FALSE, FALSE, FALSE, FALSE, FALSE, FALSE, FALSE, FALSE, FALSE, FALSE, FALSE, FALSE, FALSE, FALSE], [FALSE, FALSE, FALSE, FALSE, FALSE, FALSE, FALSE, FALSE, FALSE, FALSE, FALSE, FALSE, FALSE, FALSE, FALSE, FALSE], [FALSE, FALSE, FALSE, FALSE, FALSE, FALSE, FALSE, FALSE, FALSE, FALSE, FALSE, FALSE, FALSE, FALSE, FALSE, FALSE], [FALSE, FALSE, FALSE, FALSE, FALSE, FALSE, FALSE, FALSE, FALSE, FALSE, FALSE, FALSE, FALSE, FALSE, FALSE, FALSE], [FALSE, FALSE, FALSE, FALSE, FALSE, FALSE, FALSE, FALSE, FALSE, FALSE, FALSE, FALSE, FALSE, FALSE, FALSE, FALSE], [FALSE, FALSE, FALSE, FALSE, FALSE, FALSE, FALSE, FALSE, FALSE, FALSE, FALSE, FALSE, FALSE, FALSE, FALSE, FALSE], [FALSE, FALSE, FALSE, FALSE, FALSE, FALSE, FALSE, FALSE, FALSE, FALSE, FALSE, FALSE, FALSE, FALSE, FALSE, FALSE], [FALSE, FALSE, FALSE, FALSE, FALSE, FALSE, FALSE, FALSE, FALSE, FALSE, FALSE, FALSE, FALSE, FALSE, FALSE, FALSE], [FALSE, FALSE, FALSE, FALSE, FALSE, FALSE, FALSE, FALSE, FALSE, FALSE, FALSE, FALSE, FALSE, FALSE, FALSE, FALSE], [FALSE, FALSE, FALSE, FALSE, FALSE, FALSE, FALSE, FALSE, FALSE, FALSE, FALSE, FALSE, FALSE, FALSE, FALSE, FALSE], [FALSE, FALSE, FALSE, FALSE, FALSE, FALSE, FALSE, FALSE, FALSE, FALSE, FALSE, FALSE, FALSE, FALSE, FALSE, FALSE], [FALSE, FALSE, FALSE, FALSE, FALSE, FALSE, FALSE, FALSE, FALSE, FALSE, FALSE, FALSE, FALSE, FALSE, FALSE, FALSE], [FALSE, FALSE, FALSE, FALSE, FALSE, FALSE, FALSE, FALSE, FALSE, FALSE, FALSE, FALSE, FALSE, FALSE, FALSE, FALSE], [FALSE, FALSE, FALSE, FALSE, FALSE, FALSE, FALSE, FALSE, FALSE, FALSE, FALSE, FALSE, FALSE, FALSE, FALSE, FALSE], [FALSE, FALSE, FALSE, FALSE, FALSE, FALSE, FALSE, FALSE, FALSE, FALSE, FALSE, FALSE, FALSE, FALSE, FALSE, FALSE], [FALSE, FALSE, FALSE, FALSE, FALSE, FALSE, FALSE, FALSE, FALSE, FALSE, FALSE, FALSE, FALSE, FALSE, FALSE, FALSE], [FALSE, FALSE, FALSE, FALSE, FALSE, FALSE, FALSE, FALSE, FALSE, FALSE, FALSE, FALSE, FALSE, FALSE, FALSE, FALSE], [FALSE, FALSE, FALSE, FALSE, FALSE, FALSE, FALSE, FALSE, FALSE, FALSE, FALSE, FALSE, FALSE, FALSE, FALSE, FALSE], [FALSE, FALSE, FALSE, FALSE, FALSE, FALSE, FALSE, FALSE, FALSE, FALSE, FALSE, FALSE, FALSE, FALSE, FALSE, FALSE], [FALSE, FALSE, FALSE, FALSE, FALSE, FALSE, FALSE, FALSE, FALSE, FALSE, FALSE, FALSE, FALSE, FALSE, FALSE, FALSE], [FALSE, FALSE, FALSE, FALSE, FALSE, FALSE, FALSE, FALSE, FALSE, FALSE, FALSE, FALSE, FALSE, FALSE, FALSE, FALSE], [FALSE, FALSE, FALSE, FALSE, FALSE, FALSE, FALSE, FALSE, FALSE, FALSE, FALSE, FALSE, FALSE, FALSE, FALSE, FALSE], [FALSE, FALSE, FALSE, FALSE, FALSE, FALSE, FALSE, FALSE, FALSE, FALSE, FALSE, FALSE, FALSE, FALSE, FALSE, FALSE], [FALSE, FALSE, FALSE, FALSE, FALSE, FALSE, FALSE, FALSE, FALSE, FALSE, FALSE, FALSE, FALSE, FALSE, FALSE, FALSE], [FALSE, FALSE, FALSE, FALSE, FALSE, FALSE, FALSE, FALSE, FALSE, FALSE, FALSE, FALSE, FALSE, FALSE, FALSE, FALSE], [FALSE, FALSE, FALSE, FALSE, FALSE, FALSE, FALSE, FALSE, FALSE, FALSE, FALSE, FALSE, FALSE, FALSE, FALSE, FALSE], [FALSE, FALSE, FALSE, FALSE, FALSE, FALSE, FALSE, FALSE, FALSE, FALSE, FALSE, FALSE, FALSE, FALSE, FALSE, FALSE], [FALSE, FALSE, FALSE, FALSE, FALSE, FALSE, FALSE, FALSE, FALSE, FALSE, FALSE, FALSE, FALSE, FALSE, FALSE, FALSE], [FALSE, FALSE, FALSE, FALSE, FALSE, FALSE, FALSE, FALSE, FALSE, FALSE, FALSE, FALSE, FALSE, FALSE, FALSE, FALSE], [FALSE, FALSE, FALSE, FALSE, FALSE, FALSE, FALSE, FALSE, FALSE, FALSE, FALSE, FALSE, FALSE, FALSE, FALSE, FALSE], [FALSE, FALSE, FALSE, FALSE, FALSE, FALSE, FALSE, FALSE, FALSE, FALSE, FALSE, FALSE, FALSE, FALSE, FALSE, FALSE], [FALSE, FALSE, FALSE, FALSE, FALSE, FALSE, FALSE, FALSE, FALSE, FALSE, FALSE, FALSE, FALSE, FALSE, FALSE, FALSE], [FALSE, FALSE, FALSE, FALSE, FALSE, FALSE, FALSE, FALSE, FALSE, FALSE, FALSE, FALSE, FALSE, FALSE, FALSE, FALSE], [FALSE, FALSE, FALSE, FALSE, FALSE, FALSE, FALSE, FALSE, FALSE, FALSE, FALSE, FALSE, FALSE, FALSE, FALSE, FALSE], [FALSE, FALSE, FALSE, FALSE, FALSE, FALSE, FALSE, FALSE, FALSE, FALSE, FALSE, FALSE, FALSE, FALSE, FALSE, FALSE], [FALSE, FALSE, FALSE, FALSE, FALSE, FALSE, FALSE, FALSE, FALSE, FALSE, FALSE, FALSE, FALSE, FALSE, FALSE, FALSE], [FALSE, FALSE, FALSE, FALSE, FALSE, FALSE, FALSE, FALSE, FALSE, FALSE, FALSE, FALSE, FALSE, FALSE, FALSE, FALSE], [FALSE, FALSE, FALSE, FALSE, FALSE, FALSE, FALSE, FALSE, FALSE, FALSE, FALSE, FALSE, FALSE, FALSE, FALSE, FALSE], [FALSE, FALSE, FALSE, FALSE, FALSE, FALSE, FALSE, FALSE, FALSE, FALSE, FALSE, FALSE, FALSE, FALSE, FALSE, FALSE], [FALSE, FALSE, FALSE, FALSE, FALSE, FALSE, FALSE, FALSE, FALSE, FALSE, FALSE, FALSE, FALSE, FALSE, FALSE, FALSE], [FALSE, FALSE, FALSE, FALSE, FALSE, FALSE, FALSE, FALSE, FALSE, FALSE, FALSE, FALSE, FALSE, FALSE, FALSE, FALSE], [FALSE, FALSE, FALSE, FALSE, FALSE, FALSE, FALSE, FALSE, FALSE, FALSE, FALSE, FALSE, FALSE, FALSE, FALSE, FALSE], [FALSE, FALSE, FALSE, FALSE, FALSE, FALSE, FALSE, FALSE, FALSE, FALSE, FALSE, FALSE, FALSE, FALSE, FALSE, FALSE], [FALSE, FALSE, FALSE, FALSE, FALSE, FALSE, FALSE, FALSE, FALSE, FALSE, FALSE, FALSE, FALSE, FALSE, FALSE, FALSE], [FALSE, FALSE, FALSE, FALSE, FALSE, FALSE, FALSE, FALSE, FALSE, FALSE, FALSE, FALSE, FALSE, FALSE, FALSE, FALSE], [FALSE, FALSE, FALSE, FALSE, FALSE, FALSE, FALSE, FALSE, FALSE, FALSE, FALSE, FALSE, FALSE, FALSE, FALSE, FALSE], [FALSE, FALSE, FALSE, FALSE, FALSE, FALSE, FALSE, FALSE, FALSE, FALSE, FALSE, FALSE, FALSE, FALSE, FALSE, FALSE], [FALSE, FALSE, FALSE, FALSE, FALSE, FALSE, FALSE, FALSE, FALSE, FALSE, FALSE, FALSE, FALSE, FALSE, FALSE, FALSE], [FALSE, FALSE, FALSE, FALSE, FALSE, FALSE, FALSE, FALSE, FALSE, FALSE, FALSE, FALSE, FALSE, FALSE, FALSE, FALSE], [FALSE, FALSE, FALSE, FALSE, FALSE, FALSE, FALSE, FALSE, FALSE, FALSE, FALSE, FALSE, FALSE, FALSE, FALSE, FALSE], [FALSE, FALSE, FALSE, FALSE, FALSE, FALSE, FALSE, FALSE, FALSE, FALSE, FALSE, FALSE, FALSE, FALSE, FALSE, FALSE], [FALSE, FALSE, FALSE, FALSE, FALSE, FALSE, FALSE, FALSE, FALSE, FALSE, FALSE, FALSE, FALSE, FALSE, FALSE, FALSE], [FALSE, FALSE, FALSE, FALSE, FALSE, FALSE, FALSE, FALSE, FALSE, FALSE, FALSE, FALSE, FALSE, FALSE, FALSE, FALSE], [FALSE, FALSE, FALSE, FALSE, FALSE, FALSE, FALSE, FALSE, FALSE, FALSE, FALSE, FALSE, FALSE, FALSE, FALSE, FALSE], [FALSE, FALSE, FALSE, FALSE, FALSE, FALSE, FALSE, FALSE, FALSE, FALSE, FALSE, FALSE, FALSE, FALSE, FALSE, FALSE], [FALSE, FALSE, FALSE, FALSE, FALSE, FALSE, FALSE, FALSE, FALSE, FALSE, FALSE, FALSE, FALSE, FALSE, FALSE, FALSE], [FALSE, FALSE, FALSE, FALSE, FALSE, FALSE, FALSE, FALSE, FALSE, FALSE, FALSE, FALSE, FALSE, FALSE, FALSE, FALSE], [FALSE, FALSE, FALSE, FALSE, FALSE, FALSE, FALSE, FALSE, FALSE, FALSE, FALSE, FALSE, FALSE, FALSE, FALSE, FALSE], [FALSE, FALSE, FALSE, FALSE, FALSE, FALSE, FALSE, FALSE, FALSE, FALSE, FALSE, FALSE, FALSE, FALSE, FALSE, FALSE], [FALSE, FALSE, FALSE, FALSE, FALSE, FALSE, FALSE, FALSE, FALSE, FALSE, FALSE, FALSE, FALSE, FALSE, FALSE, FALSE], [FALSE, FALSE, FALSE, FALSE, FALSE, FALSE, FALSE, FALSE, FALSE, FALSE, FALSE, FALSE, FALSE, FALSE, FALSE, FALSE], [FALSE, FALSE, FALSE, FALSE, FALSE, FALSE, FALSE, FALSE, FALSE, FALSE, FALSE, FALSE, FALSE, FALSE, FALSE, FALSE], [FALSE, FALSE, FALSE, FALSE, FALSE, FALSE, FALSE, FALSE, FALSE, FALSE, FALSE, FALSE, FALSE, FALSE, FALSE, FALSE], [FALSE, FALSE, FALSE, FALSE, FALSE, FALSE, FALSE, FALSE, FALSE, FALSE, FALSE, FALSE, FALSE, FALSE, FALSE, FALSE], [FALSE, FALSE, FALSE, FALSE, FALSE, FALSE, FALSE, FALSE, FALSE, FALSE, FALSE, FALSE, FALSE, FALSE, FALSE, FALSE], [FALSE, FALSE, FALSE, FALSE, FALSE, FALSE, FALSE, FALSE, FALSE, FALSE, FALSE, FALSE, FALSE, FALSE, FALSE, FALSE], [FALSE, FALSE, FALSE, FALSE, FALSE, FALSE, FALSE, FALSE, FALSE, FALSE, FALSE, FALSE, FALSE, FALSE, FALSE, FALSE], [FALSE, FALSE, FALSE, FALSE, FALSE, FALSE, FALSE, FALSE, FALSE, FALSE, FALSE, FALSE, FALSE, FALSE, FALSE, FALSE], [FALSE, FALSE, FALSE, FALSE, FALSE, FALSE, FALSE, FALSE, FALSE, FALSE, FALSE, FALSE, FALSE, FALSE, FALSE, FALSE], [FALSE, FALSE, FALSE, FALSE, FALSE, FALSE, FALSE, FALSE, FALSE, FALSE, FALSE, FALSE, FALSE, FALSE, FALSE, FALSE], [FALSE, FALSE, FALSE, FALSE, FALSE, FALSE, FALSE, FALSE, FALSE, FALSE, FALSE, FALSE, FALSE, FALSE, FALSE, FALSE], [FALSE, FALSE, FALSE, FALSE, FALSE, FALSE, FALSE, FALSE, FALSE, FALSE, FALSE, FALSE, FALSE, FALSE, FALSE, FALSE]] ("Boolean array 2"), Variant=w127) -> (data=w124:bool[][], error out=w122:errorcluster)
            n29 = Bundle By Name(cluster=w125, "Boolean array"=w124) -> (w121:T1)
          }
          frame "KEYENCE Marking Compl Clear" {
            n30 = Variant To Data(error in=w143, type=TRUE, Variant=w144) -> (data=w130:bool, error out=w140:errorcluster)
            n31 = Bundle By Name(cluster=w134, "Control.Marking Compl Clear"=w130) -> (w132:T1)
            n32 = Unbundle By Name(w132) -> ("Communication Opened"=w133:bool, "Control"=w135:T3, "Ethernet/IP parameters.Network path"=w139:string, "Ethernet/IP parameters.Class"=w138:dbl, "Ethernet/IP parameters.Set Instance"=w137:dbl, "Ethernet/IP parameters.Attribute"=w136:dbl)
            n33 = case shown="True" w133 {
              tunnel: [w145 w147] -> w141
              tunnel: w140 -> [w145 w155]
              tunnel: w139 -> [_ w154]
              tunnel: w138 -> [_ w153]
              tunnel: w137 -> [_ w152]
              tunnel: w136 -> [_ w151]
              tunnel: w135 -> [_ w150]
              tunnel: w132 -> [w146 w148]
              tunnel: [w146 w148] -> w131
              tunnel: w130 -> [_ _]
              tunnel: w129 -> [_ _]
              frame False {
              }
              frame True {
                n34 = call "SetControl_EIP.vi"("variant"=w150) -> ("Data"=w149:u8[])  [unwired: 10 in]
                n35 = call <vilib>:"EthernetIP CIP Set Attribute Single.vi"("Network Path"=w154, "Data"=w149, "error in"=w155, "Class"=w153, "Instance"=w152, "Attribute"=w151) -> ("error out"=w147:errorcluster)  [unwired: 8 in, 1 out]
              }
            }
          }
          frame "KEYENCE Error clear" {
            n36 = Variant To Data(error in=w170, type=TRUE, Variant=w171) -> (data=w163:bool, error out=w167:errorcluster)
            n37 = Bundle By Name(cluster=w162, "Control.Error clear"=w163) -> (w160:T1)
            n38 = Unbundle By Name(w160) -> ("Communication Opened"=w161:bool, "Control"=w164:T3, "Ethernet/IP parameters.Network path"=w166:string, "Ethernet/IP parameters.Class"=w165:dbl, "Boolean array"=w156:bool[][])  [unwired: 2 out]
            n39 = case shown="True" w161 {
              tunnel: [w173 w182] -> w168
              tunnel: w167 -> [w173 w178]
              tunnel: w166 -> [_ w181]
              tunnel: w165 -> [_ _]
              tunnel: w164 -> [_ w185]
              tunnel: w160 -> [w174 w184]
              tunnel: [w174 w184] -> w159
              tunnel: w158 -> [w172 w176]
              tunnel: [w172 w175] -> w157
              tunnel: w156 -> [_ w183]
              frame False {
              }
              frame True {
                n40 = call "SetControl_EIP.vi"("Boolean array 2"=w183, "variant"=w185) -> ()  [unwired: 9 in, 1 out]
                n41 = call-poly <vilib>:"EthernetIP Tag Write.vi"("Session in"=w176, "Network Path"=w181, "Tag Name"="Error Clear", "Data"=bool[] [TRUE], "error in"=w178) -> ("Session out"=w175:T5, "error out"=w177:errorcluster)  [unwired: 9 in]
                n42 = call <vilib>:"Clear Errors.vi"("error in (no error)"=w177) -> ("error out"=w182:errorcluster)  [unwired: 5 in, 1 out]
              }
            }
          }
          frame "KEYENCE Error Clear Compl Clear" {
            n43 = Variant To Data(error in=w201, type=TRUE, Variant=w202) -> (data=w188:bool, error out=w198:errorcluster)
            n44 = Bundle By Name(cluster=w192, "Control.Error Clear Compl Clear"=w188) -> (w190:T1)
            n45 = Unbundle By Name(w190) -> ("Communication Opened"=w191:bool, "Control"=w193:T3, "Ethernet/IP parameters.Network path"=w197:string, "Ethernet/IP parameters.Class"=w196:dbl, "Ethernet/IP parameters.Set Instance"=w195:dbl, "Ethernet/IP parameters.Attribute"=w194:dbl)
            n46 = case shown="True" w191 {
              tunnel: [w203 w205] -> w199
              tunnel: w198 -> [w203 w213]
              tunnel: w197 -> [_ w212]
              tunnel: w196 -> [_ w211]
              tunnel: w195 -> [_ w210]
              tunnel: w194 -> [_ w209]
              tunnel: w193 -> [_ w208]
              tunnel: w190 -> [w204 w206]
              tunnel: [w204 w206] -> w189
              tunnel: w188 -> [_ _]
              tunnel: w187 -> [_ _]
              frame False {
              }
              frame True {
                n47 = call "SetControl_EIP.vi"("variant"=w208) -> ("Data"=w207:u8[])  [unwired: 10 in]
                n48 = call <vilib>:"EthernetIP CIP Set Attribute Single.vi"("Network Path"=w212, "Data"=w207, "error in"=w213, "Class"=w211, "Instance"=w210, "Attribute"=w209) -> ("error out"=w205:errorcluster)  [unwired: 8 in, 1 out]
              }
            }
          }
          frame "KEYENCE Program Change" {
            n49 = Variant To Data(error in=w229, type=u16 0, Variant=w230) -> (data=w217:u16, error out=w228:errorcluster)
            n50 = Bundle By Name(cluster=w222, "Status.Program No"=w217) -> (w220:T1)
            n51 = Unbundle By Name(w220) -> ("Communication Opened"=w221:bool, "Control"=w223:T3, "Ethernet/IP parameters.Network path"=w227:string, "Ethernet/IP parameters.Class"=w226:dbl, "Ethernet/IP parameters.Set Instance"=w225:dbl, "Ethernet/IP parameters.Attribute"=w224:dbl)
            n52 = case shown="True" w221 {
              tunnel: [w232 w243] -> w215
              tunnel: w228 -> [w232 w242]
              tunnel: w227 -> [_ w241]
              tunnel: w226 -> [_ w240]
              tunnel: w225 -> [_ w239]
              tunnel: w224 -> [_ w238]
              tunnel: w223 -> [_ w237]
              tunnel: w220 -> [w233 w235]
              tunnel: [w233 w235] -> w219
              tunnel: w216 -> [w231 w234]
              tunnel: [w231 w234] -> _
              frame False {
              }
              frame True {
                n53 = call "SetControl_EIP.vi"("variant"=w237) -> ("Data"=w236:u8[])  [unwired: 10 in]
                n54 = call <vilib>:"EthernetIP CIP Set Attribute Single.vi"("Network Path"=w241, "Data"=w236, "error in"=w242, "Class"=w240, "Instance"=w239, "Attribute"=w238) -> ("error out"=w243:errorcluster)  [unwired: 8 in, 1 out]
              }
            }
          }
          frame "KEYENCE Program Change 2" {
            n55 = Variant To Data(error in=w259, type=TRUE, Variant=w260) -> (data=w245:bool, error out=w257:errorcluster)
            n56 = Bundle By Name(cluster=w251, "Control.Program Change"=w245) -> (w249:T1)
            n57 = Unbundle By Name(w249) -> ("Communication Opened"=w250:bool, "Control"=w252:T3, "Ethernet/IP parameters.Network path"=w256:string, "Ethernet/IP parameters.Class"=w255:dbl, "Ethernet/IP parameters.Set Instance"=w254:dbl, "Ethernet/IP parameters.Attribute"=w253:dbl)
            n58 = case shown="True" w250 {
              tunnel: [w261 w263] -> w258
              tunnel: w257 -> [w261 w271]
              tunnel: w256 -> [_ w270]
              tunnel: w255 -> [_ w269]
              tunnel: w254 -> [_ w268]
              tunnel: w253 -> [_ w267]
              tunnel: w252 -> [_ w266]
              tunnel: w249 -> [w262 w264]
              tunnel: [w262 w264] -> w248
              tunnel: w246 -> [_ _]
              tunnel: w245 -> [_ _]
              frame False {
              }
              frame True {
                n59 = call "SetControl_EIP.vi"("variant"=w266) -> ("Data"=w265:u8[])  [unwired: 10 in]
                n60 = call <vilib>:"EthernetIP CIP Set Attribute Single.vi"("Network Path"=w270, "Data"=w265, "error in"=w271, "Class"=w269, "Instance"=w268, "Attribute"=w267) -> ("error out"=w263:errorcluster)  [unwired: 8 in, 1 out]
              }
            }
          }
          frame "KEYENCE Program Change Compl Clear" {
            n61 = Variant To Data(error in=w287, type=TRUE, Variant=w288) -> (data=w274:bool, error out=w284:errorcluster)
            n62 = Bundle By Name(cluster=w278, "Control.Program Change Compl Clear"=w274) -> (w276:T1)
            n63 = Unbundle By Name(w276) -> ("Communication Opened"=w277:bool, "Control"=w279:T3, "Ethernet/IP parameters.Network path"=w283:string, "Ethernet/IP parameters.Class"=w282:dbl, "Ethernet/IP parameters.Set Instance"=w281:dbl, "Ethernet/IP parameters.Attribute"=w280:dbl)
            n64 = case shown="True" w277 {
              tunnel: [w289 w291] -> w285
              tunnel: w284 -> [w289 w299]
              tunnel: w283 -> [_ w298]
              tunnel: w282 -> [_ w297]
              tunnel: w281 -> [_ w296]
              tunnel: w280 -> [_ w295]
              tunnel: w279 -> [_ w294]
              tunnel: w276 -> [w290 w292]
              tunnel: [w290 w292] -> w275
              tunnel: w274 -> [_ _]
              tunnel: w273 -> [_ _]
              frame False {
              }
              frame True {
                n65 = call "SetControl_EIP.vi"("variant"=w294) -> ("Data"=w293:u8[])  [unwired: 10 in]
                n66 = call <vilib>:"EthernetIP CIP Set Attribute Single.vi"("Network Path"=w298, "Data"=w293, "error in"=w299, "Class"=w297, "Instance"=w296, "Attribute"=w295) -> ("error out"=w291:errorcluster)  [unwired: 8 in, 1 out]
              }
            }
          }
          frame "Abort" {
            n67 = Flush Queue(queue=w303, error in (no error)=w304) -> (error out=w301:errorcluster)  [unwired: 2 out]
          }
          frame "Error" {
            n68 = Unbundle By Name(w309) -> ("UI"=w314:refnum<queue>)
            n69 = call-poly "Enqueue Message.vi"("error in (no error)"=w307, "Message Data"=w308, "Message"="Error", "Message Queue"=w314) -> ("error out"=w316:errorcluster)  [unwired: 6 in, 1 out]
            n70 = call-poly "Enqueue Message.vi"("Priority Message? (F)"=TRUE, "error in (no error)"=w307, "Message"="Initiate Stop", "Message Queue"=w310) -> ("error out"=w315:errorcluster)  [unwired: 6 in, 1 out]
            n71 = Merge Errors(w316, w315) -> (w311:errorcluster)
          }
          frame "Initiate Stop" {
            n72 = call-poly "Enqueue Message.vi"("Priority Message? (F)"=TRUE, "error in (no error)"=w322, "Message"="Program Stop", "Message Queue"=w321) -> ("error out"=w323:errorcluster)  [unwired: 6 in, 1 out]
          }
          frame "Program Stop" {
            n73 = Flush Queue(queue=w336, error in (no error)=w326) -> (error out=w328:errorcluster)  [unwired: 2 out]
            n74 = Unbundle By Name(w329) -> ("Keyence Data"=w330:refnum<queue>)
            n75 = Flush Queue(queue=w330, error in (no error)=w326) -> (queue out=w331:refnum<queue>, error out=w332:errorcluster)  [unwired: 1 out]
            n76 = Release Queue(queue=w331, error in (no error)=w332) -> (error out=w333:errorcluster)  [unwired: 1 in, 2 out]
            n77 = Merge Errors(w333, w328) -> (w327:errorcluster)
          }
          frame Default {
            n78 = xnode "Error Ring"("parameter 0"=w338) -> ("error out"=w339:errorcluster)
          }
        }
      }
      frame True {
        n79 = Unbundle By Name(w362) -> ("Boolean array"=w351:bool[][], "Control"=w353:T3, "Communication Opened"=w357:bool, "Ethernet/IP parameters.Network path"=w361:string, "Ethernet/IP parameters.Class"=w360:dbl, "Ethernet/IP parameters.Get Instance"=w359:dbl, "Ethernet/IP parameters.Attribute"=w358:dbl, "Ethernet/IP parameters.Set Instance"=w352:dbl)  [unwired: 1 out]
        n80 = Unbundle By Name(w356) -> ("Keyence Data"=w355:refnum<queue>)
        n81 = case shown="True" w357 {
          tunnel: [w367 w392] -> w364
          tunnel: w363 -> [w368 w384]
          tunnel: w362 -> [w369 w391]
          tunnel: w361 -> [_ w385]
          tunnel: w360 -> [_ _]
          tunnel: w359 -> [_ _]
          tunnel: w358 -> [_ _]
          tunnel: w355 -> [w370 w388]
          tunnel: [w369 w387] -> w354
          tunnel: w353 -> [_ w386]
          tunnel: w352 -> [_ _]
          tunnel: w351 -> [_ w382]
          tunnel: w350 -> [w366 w372]
          tunnel: [w366 w372] -> w349
          frame False {
            n82 = call-poly "Lossy Enqueue Message.vi"("error in (no error)"=w368, "Message Data"=w369, "Message"="Keyence Data", "Message Queue"=w370) -> ("error out"=w367:errorcluster)  [unwired: 6 in, 1 out]
          }
          frame True {
            n83 = disable-structure shown="Disabled" {
              disable-tunnel: w386 -> [w404 _]
              disable-tunnel: w385 -> [w403 _]
              disable-tunnel: w384 -> [w401 _]
              disable-tunnel: "Attribute" -> [w400 _]
              disable-tunnel: w382 -> [w398 _]
              disable-tunnel: [w396 _] -> w380
              disable-tunnel: "Class" -> [w395 _]
              disable-tunnel: "Inst" -> [w394 _]
              frame Disabled {
                n84 = call "SetControl_EIP.vi"(7:TRUE ("select"), "Boolean array 2"=w398, "variant"=w404) -> ("Data"=w405:u8[])  [unwired: 8 in]
                n85 = call <vilib>:"EthernetIP CIP Set Attribute Single.vi"("Timeout (ms)"=1000, "Network Path"=w403, "Data"=w405, "error in"=w401, "Class"=w395, "Instance"=w394, "Attribute"=w400) -> ("error out"=w397:errorcluster)  [unwired: 7 in, 1 out]
                n86 = call <vilib>:"Clear Errors.vi"("error in (no error)"=w397) -> ("error out"=w396:errorcluster)  [unwired: 5 in, 1 out]
              }
              frame Enabled {
              }
            }
            n87 = call <vilib>:"EthernetIP CIP Get Attribute Single.vi"("Timeout (ms)"=1000, "Network Path"=w385, "error in"=w380, "Class"="Class 2", "Instance"="Inst 2", "Attribute"="Attribute 2") -> ("Data"=w390:u8[], "error out"=w379:errorcluster)  [unwired: 7 in, 1 out]
            n88 = call "GetStatus_EIP.vi"("Data"=w390) -> ("Status"=w389:T7)  [unwired: 10 in]
            n89 = call <vilib>:"Clear Errors.vi"("error in (no error)"=w379) -> ("error out"=w378:errorcluster)  [unwired: 5 in, 1 out]
            n90 = Bundle By Name(cluster=w391, "Status"=w389) -> (w387:T1)
            n91 = call-poly "Lossy Enqueue Message.vi"("error in (no error)"=w378, "Message Data"=w387, "Message"="Keyence Data", "Message Queue"=w388) -> ("error out"=w392:errorcluster)  [unwired: 6 in, 1 out]
          }
        }
      }
    }
    "Keyence Data Cluster" <- w10
    n92 = call "Error Handler - Message Handling Loop.vi"("error in (no error)"=w14, "Message Queue"=w11) -> ("dup error in"=w15:errorcluster, "dup Message Queue"=w12:refnum<queue>)  [unwired: 8 in]
  }
  "error out" <- w7
  "Message Queue" <- w3
